vi "MAIN - PECT - Autonics - Pulses - encoder - stm32.vi"() -> ()   [LabVIEW 2018]
uses:
  Control 1.ctl
  <vilib>/DAQmx/read.llb/DAQmx Read (Counter U32 1Chan 1Samp).vi
  <vilib>/DAQmx/write.llb/DAQmx Write (Analog 1D Wfm NChan NSamp).vi
  <vilib>/DAQmx/read.llb/DAQmx Read (Analog 1D Wfm NChan NSamp).vi
  <vilib>/Instr/_visa.llb/VISA Configure Serial Port (Instr).vi
  <vilib>/DAQmx/create/channels.llb/DAQmx Create Channel (AI-Voltage-Basic).vi
  <vilib>/DAQmx/create/channels.llb/DAQmx Create Channel (CI-Count Edges).vi
  <vilib>/DAQmx/miscellaneous.llb/DAQmx Fill In Error Info.vi
  <vilib>/DAQmx/configure/timing.llb/DAQmx Timing (Sample Clock).vi
  <vilib>/DAQmx/configure/trigger.llb/DAQmx Start Trigger (Digital Edge).vi
  <vilib>/DAQmx/create/channels.llb/DAQmx Create Channel (AO-Voltage-Basic).vi
  LabViewtoPython/Global_data.vi
  <vilib>/measure/maspectr.llb/FFT Power Spectrum and PSD for 1 Chan.vi
  <resource>/objmgr/daqmx.rc
  <vilib>/Platform/NI_3dgraph.lvlib
  <vilib>/measure/NI_MAPro.lvlib
panel:
  in  "Filter 2":bool
  in  "low cutoff freq: fl 2":dbl=40.0 format="%0.2f"
  in  "Backdata":bool
  out "Numeric 2":i32=7858
  out "Init pulses":i32
  in  "Motor counter":tag="Dev3/ctr0"
  in  "Motor Counter Terminal":tag="PFI8"
  out "dy":dbl[][](array[numeric])
  in  "2D Array In":dbl[][](array[numeric])
  out "Output":dbl[][](array[numeric])
  out "Current  Position (mm)":dbl=12.5
  out "Acquire":bool=TRUE
  out "Numeric":dbl=22.0
  out "Enum":T1(ring)
  in  "Direction (+)":string="+"
  in  "Tab Control 3":enum32{"Control", "Data Processing"}(tab)
  in  "Encoder":bool=TRUE
  in  "Home":bool
  in  "Exit":bool
  in  "Scan":bool
  in  "Move Dis(mm)":dbl=150.0
  in  "Right":bool
  in  "Forward":bool
  in  "Left":bool
  in  "Backward":bool
  in  "Stop":bool
  in  "Pulser Trigger":tag="/Dev3/PFI0"
  in  "Edge":i32(ring)=10280 items=["Rising"=10280, "Falling"=10171]
  in  "2 Plots":bool
  in  "Offset":bool
  in  "Open csv":bool
  in  "Save Scan mode":bool caption="Save Process"
  in  "Gate 1":dbl
  in  "Gate 2":dbl=20.0
  in  "Open tdms":bool
  in  "Tab Control 4":enum32{"Basic", "Gaussian", "Chirp"}(tab)
  in  "Pulse Basic":T3={"Basic amp"=8.0, "Duty cycle %"=50.0, "Basic freq (Hz)"=200, "Basic Type"=2} {"Basic Type" items=["Sine Wave", "Triangle Wave", "Square Wave", "Sawtooth Wave"]; "Duty cycle %" format="%#.2f"; "Basic amp" format="%0.2p"}
  in  "Pulse Gaussian":T4={"Gauss amp"=2.8, "Gauss Nor. Band"=0.5, "Gauss atten (dB)"=6.0, "Gauss freq (Hz)"=1000.0}
  in  "Pulse chirp":T5={"Chirp amp"=2.1, "Chirp f2"=1500.0, "Chirp f1"=500.0} {"Chirp f1" format="%0.2f"; "Chirp f2" format="%0.2f"; "Chirp amp" format="%0.2f"}
  out "Motor Pulses":i32
  in  "Start idx":i32
  in  "End idx":i32=2000
  in  "Cursor":bool=TRUE
  in  "Repair Line Col":bool
  in  "Repair Line Row":bool
  in  "Line Col":dbl=167.0
  in  "Line Row":dbl
  in  "Y-max":dbl=55.0
  in  "Y-min":dbl
  in  "X-max":dbl=319.0
  in  "X-min":dbl
  in  "Inverse":bool caption="Scan"
  in  "ViewMode":i32(ring) items=["cwViewXYPlane", "cwViewXZPlane", "cwViewYZPlane", "cwViewUserDefined"]
  in  "Plot style":i32(ring)=5 items=["cwLine"=1, "cwPoint"=2, "cwLinePoint"=3, "cwHiddenLine"=4, "cwSurface"=5, "cwSurfaceLine"=6, "cwSurfaceNormal"=7, "cwContourLine"=8, "cwSurfaceContour"=9]
  in  "ColorMapAutoScale":bool=TRUE
  in  "Max":dbl=0.6
  in  "Min":dbl=-0.8
  in  "low cutoff freq: fl":dbl=40.0 format="%0.2f"
  in  "Filter":bool caption="Scan"
  in  "Backindex":i32
  in  "Backdata":bool caption="Scan"
  in  "Odd":bool caption="Scan"
  in  "DiffX":bool caption="Scan"
  in  "DiffY":bool caption="Scan"
  in  "Abs":bool caption="Scan"
  in  "Trim data":bool caption="Scan"
  in  "Return":bool caption="Scan"
  out "No.data":i32
  in  "Tab Control 2":T6(tab)
  out "Hall sensors signal":waveform(dbl)[](graph)=[{"t0"=timestamp(3772601412.9474645 s since 1904-01-01), "dt"=9.999999999999972e-06, "Y"=array[500 elements], "attributes"=variant("NI_ChannelName"=variant(string "Acquisition Task0"), "NI_UnitDescription"=variant(string "Volts"))}, {"t0"=timestamp(3772601412.9474645 s since 1904-01-01), "dt"=9.999999999999972e-06, "Y"=array[500 elements], "attributes"=variant("NI_ChannelName"=variant(string "Acquisition Task0"), "NI_UnitDescription"=variant(string "Volts"))}]
  out "Feature Extraction":dbl(graph)=9.808813079931117
  out "Power spectral density":cluster{"f0":dbl, "df":dbl, "magnitude":dbl[]}[](graph)=[{"f0"=0.0, "df"=200.00000000000054, "magnitude"=[0.014362964529831107, 8.310174695746657, 3.5091233603848444, 0.7631604563682475, 0.42177215625270154, 0.19736118568021033, 0.12192952566419618, 0.06836206987142136, 0.04491682851594746, 0.027429593107677796, 0.018839071574379328, 0.012148402422180482, 0.00862941575502791, 0.005816349612651425, 0.004256233122154165, 0.0029703985982499756, 0.00222866785183307, 0.001605169236331863, 0.0012333117661796167, 0.0009173667056733339, 0.0007155423005092866, 0.0005404107405385125, 0.00042969027524349985, 0.000330389538775732, 0.00026610143624204957, 0.00021016892953679833, 0.00017149707496417528, 0.0001376562085986954, 0.00011376018152653006, 9.192625603438476e-05, 7.690968629569889e-05, 6.331696380512943e-05, 5.369944415943588e-05, 4.483264313157133e-05, 3.783661085972104e-05, 3.171641922275525e-05, 2.7287859659355045e-05, 2.2939811822779873e-05, 1.9729023645397208e-05, 1.6853998605376913e-05, 1.4418164836398328e-05, 1.2221148062729234e-05, 1.0824528543421417e-05, 9.63348776166626e-06, 8.38664900977408e-06, 7.088182653208775e-06, 6.4216695750381725e-06, 5.838100076590925e-06, 5.062973197813572e-06, 4.380481399910079e-06, 4.008311134417931e-06, 3.567777110785873e-06, 3.1057220585572244e-06, 2.7147559678671816e-06, 2.469004683700486e-06, 2.2349741034633414e-06, 1.9591588689462376e-06, 1.6850457298246318e-06, 1.4830403711511327e-06, 1.2810395862247023e-06, 1.1661807691347021e-06, 1.093149967617751e-06, 1.0079255280756182e-06, 9.738198789620943e-07, 9.715762489409555e-07, 8.96196851562932e-07, 7.523554510993729e-07, 6.138187229264334e-07, 5.478503267370196e-07, 5.020387710315625e-07, 4.619114100892691e-07, 4.2419919587483664e-07, 3.871191758999957e-07, 3.3109894129644344e-07, 2.7247124240836894e-07, 2.4850669965307075e-07, 2.675581974815067e-07, 2.869535576611872e-07, 2.7749898679948705e-07, 2.4632291660033263e-07, 2.1801622453669157e-07, 1.9562127404410693e-07, 1.7794867931791103e-07, 1.6811228641885276e-07, 1.5616631012591995e-07, 1.2698956764184784e-07, 1.1852206215172555e-07, 1.4052784440882626e-07, 1.2417001647212458e-07, 1.0284765504537362e-07, 1.1149589035952914e-07, 1.0511333967341304e-07, 8.631594494061448e-08, 7.61357409684589e-08, 6.937531533687657e-08, 7.010901044974718e-08, 8.376351369143556e-08, 8.332819916917156e-08, 7.575462195169617e-08, 7.885454530850919e-08, 7.033884155079282e-08, 6.000608335599921e-08, 5.97054760945729e-08, 5.485461457908942e-08, 4.5798277681414524e-08, 3.8358139340699667e-08, 3.3676177145198874e-08, 2.359178779533516e-08, 1.8510156950926208e-07, 5.633600043987599e-07, 1.2855680539466263e-07, 1.678757147241346e-09, 9.284437562813088e-09, 1.0545287775390088e-08, 1.4885830217932153e-08, 2.288209497269105e-08, 2.873109268361236e-08, 3.240059456948882e-08, 2.9373366158461235e-08, 1.6941482060852982e-08, 1.3632670056174659e-08, 2.1599039524822428e-08, 2.864941019474429e-08, 2.6325731881126113e-08, 1.7196134685578826e-08, 1.285975985125537e-08, 2.487391402547663e-08, 3.203240697565154e-08, 1.720084880141038e-08, 1.198157151831842e-08, 4.459277430827087e-08, 3.303106142973774e-08, 2.133721419654825e-09, 5.109784879397802e-09, 1.3424442340069317e-08, 1.6867214043579696e-08, 1.5794232523657268e-08, 1.5127476306279365e-08, 1.5161128228270264e-08, 1.6118426952093236e-08, 1.68634299672962e-08, 1.6945853543588977e-08, 1.6868974698788065e-08, 1.0784883043928202e-08, 6.704461125465945e-09, 5.63854300858233e-09, 5.0266424135467835e-09, 6.568105272929862e-09, 7.59825171358279e-09, 1.1582490374347768e-08, 1.4599621166870617e-08, 1.1119981753358133e-08, 1.2942473625642193e-08, 1.774060483085851e-08, 1.2500855965824921e-08, 6.798673179813089e-09, 3.825701426335919e-09, 3.26796645153504e-09, 5.851436091197948e-09, 9.117713523866911e-09, 1.006129981484824e-08, 9.670570433095903e-09, 6.903128148171139e-09, 4.6017756529415e-09, 5.3985244057071846e-09, 5.091422999856316e-09, 6.324668231652877e-09, 1.2737016312662349e-08, 1.1044421774333567e-08, 8.651162714385546e-09, 1.1322218007796528e-08, 2.001816258965483e-08, 5.928473615592085e-09, 7.891019427142181e-08, 2.710947551074279e-08, 1.2109707937657889e-08, 1.5145237102579988e-08, 5.528097117459409e-09, 2.446227470013534e-09, 4.474934593714336e-09, 5.0407366988498425e-09, 3.111049069643071e-09, 2.815789099676651e-09, 2.198647691132389e-09, 3.564152929351252e-09, 6.267856744894125e-09, 7.855009262955687e-09, 7.797377233153132e-09, 4.960163939861098e-09, 4.126978597434626e-09, 7.818217929097502e-09, 1.2088488517836051e-08, 1.5807096200904325e-08, 1.4005329604816694e-08, 5.851220743643767e-09, 2.6117978983188714e-09, 2.109976569403879e-09, 5.079632540665155e-09, 1.4259080894475479e-08, 1.495379496959781e-08, 9.052261543456204e-09, 3.575730290321285e-09, 3.1053726421904294e-09, 4.820372466465575e-09, 4.369001562192545e-09, 3.7977013602532216e-09, 6.3454386055254605e-09, 6.575277240465807e-09, 5.475129294692274e-09, 5.322703673955227e-09, 5.009070823464934e-09, 4.896565904493876e-09, 6.143932752088867e-09, 5.958661103676973e-09, 7.581104983628496e-09, 1.29243222401234e-08, 1.639764632220392e-08, 1.62303693108852e-08, 1.4889908382954265e-08, 6.265747183052516e-09, 3.5369901111449913e-09, 3.99415669353274e-09, 4.336446347036391e-09, 5.2993261898260645e-09, 7.707397886429536e-09, 6.012570048278088e-09, 5.397447185281157e-09, 6.015860855807052e-09, 4.357450363448522e-09, 7.100715289952546e-09, 9.805560081159733e-09, 6.950732862283354e-09, 6.8841271181353234e-09, 4.007604528286423e-09, 2.256008744538429e-09, 4.9771864801295934e-09, 8.071283941533974e-09, 4.167385572741655e-09, 1.6583946978149515e-09, 4.0472343516843064e-10, 8.66146004461999e-09, 6.3560460604905285e-09, 1.133124355330132e-09, 3.296374300658255e-09, 1.0980369368354793e-08, 1.459727038058513e-08, 1.3676634631114127e-08, 8.996399934605576e-09, 6.0440593342303344e-09, 7.04368222367538e-09]}, ...(2 in all)]
  in  "Add LF":bool
  in  "Save LF":bool caption="Save Process"
  in  "3D Surface":refnum<k7>(container)
  out "Record path":path=path "G:/Shared drives/ICSLab-Students/NDT/PECT/Data/Scan NewBoard/PECT_default.tdms" caption="selected path"
  out "Feature extraction scan":dbl[](graph)
  in  "View Mode":bool caption="Scan"
  out "Hall sensors signal lf":dbl[][](graph)=[[-0.70660846198, -0.716567731313, -0.71772803455, -0.717921418426, -0.720596562008, -0.722079171705, -0.724657623384, -0.723561781416, -0.729298836376, -0.728847607304, -0.733553281611, -0.731232675116, -0.734068971955, -0.734230125187, -0.734649123582, -0.735197044564, -0.737292036575, -0.735906118769, -0.738162264033, -0.736454039766, -0.735454889741, -0.737968880154, -0.735422659102, -0.737292036581, -0.734552431644, -0.735809426849, -0.731909518652, -0.731264905752, -0.726591462081, -0.727171613726, -0.72340062815, -0.721080021693, -0.715278505501, -0.71253890069, -0.707188613582, -0.701870557272, -0.697068191179, -0.692362517146, -0.687946918849, -0.677826496722, -0.674571201711, -0.663773936246, -0.660776486438, -0.651622983945, -0.644113244288, -0.636120045089, -0.629867300614, -0.618425422989, -0.610399993434, -0.59950603696, -0.59218968167, -0.58322956384, -0.571207535404, -0.564471331877, -0.553126147145, -0.546615558225, -0.534915836753, -0.528792015616, -0.520315358066, -0.514803919133, -0.504103347861, -0.497753912499, -0.490534250062, -0.48415258421, -0.4781254554, -0.472839631231, -0.469197569495, -0.467811652195, -0.46571666097, -0.462429136198, -0.467457115235, -0.467231500771, -0.474354471106, -0.474741238726, -0.482927820085, -0.490469788806, -0.499204291135, -0.509066865834, -0.523216115386, -0.534432377128, -0.554350911396, -0.569177005115, -0.58816085171, -0.612366062487, -0.634250667901, -0.66187232831, -0.688269225307, -0.719081721676, -0.746928999864, -0.781093486223, -0.813130751347, -0.851227380515, -0.888357092222, -0.928000797226, -0.965807357181, -1.008351826422, -1.048994689492, -1.09189370194, -1.13485717869, -1.180109036257, -1.2251352826, -1.266293851833, -1.314639865003, -1.35380013893, -1.401147008934, -1.441370901989, -1.48307740981, -1.522592234217, -1.561881446939, -1.594208832793, -1.628276678402, -1.656575231322, -1.685228323683, -1.708627813295, -1.726709237842, -1.745338585167, -1.754749951221, -1.765386084343, -1.766481928394, -1.766578620469, -1.759068865834, -1.749141808352, -1.726870391409, -1.702697363978, -1.672142659225, -1.635496354594, -1.591855992024, -1.542736415895, -1.486816169566, -1.426544787201, -1.357119898907, -1.281152192711, -1.205055574576, -1.115615471107, -1.027496838527, -0.924487655795, -0.823476790057, -0.71266782326, -0.598377964549, -0.477738687781, -0.356454816131, -0.226146385508, -0.096933813379, 0.039691785785, 0.177477671952, 0.315553620416, 0.456562543074, 0.59605661768, 0.738386978448, 0.878138885599, 1.019921318004, 1.154935322631, 1.292076548544, 1.418613908244, 1.546504957955, 1.665822671713, 1.781143796386, 1.887472587349, 1.990352709737, 2.080759590593, 2.164752584475, 2.235692182322, 2.298122899903, 2.352689348501, 2.387788500997, 2.419503438832, 2.429204857999, 2.432524612792, 2.418181983039, 2.390753718718, 2.346694452024, 2.29477091497, 2.222380935278, 2.137904477937, 2.035346650361, 1.920347813654, 1.791425361517, 1.644195932762, 1.485299034053, 1.310738069287, 1.125154243505, 0.921650202866, 0.71092650171, 0.483765177519, 0.253445229601, 0.008105779367, -0.246129373952, -0.508261099919, -0.779449723152, -1.058244889529, -1.341584711586, -1.635528585329, -1.928441259944, -2.223868134907, -2.526772774422, -2.823650514512, -3.124106146674, -3.41405481644, -3.706227714753, -3.987442417835, -4.263822791101, -4.527407776882, -4.786577416573, -5.02840704592, -5.262275871216, -5.475098028081, -5.677574208879, -5.860454027961, -6.026509320014, -6.174450790588, -6.300217254762, -6.406645020668, -6.487352250666, -6.552781862445, -6.587011551361, -6.605834660103, -6.593973522799, -6.560743004097, -6.502017506172, -6.420568948967, -6.309918874295, -6.178350774499, -6.019772990024, -5.841921080871, -5.636479455639, -5.407702708707, -5.163100759281, -4.889329996495, -4.60340849308, -4.29102572782, -3.966589007543, -3.624329025262, -3.267791211866, -2.894429352616, -2.512784620922, -2.118957082525, -1.720230866355, -1.310095339563, -0.893610688781, -0.473226398891, -0.047749885035, 0.377081857903, 0.806651402224, 1.226326113266, 1.646645459066, 2.057327931374, 2.465367624173, 2.856937640696, 3.240772514315, 3.608041067282, 3.955230157274, 4.293975068757, 4.609804197942, 4.90271751193, 5.177098363499, 5.426887322034, 5.649860408204, 5.851142279943, 6.021772700426, 6.172194436626, 6.288354759714, 6.38169561436, 6.443353457295, 6.479452149573, 6.483029788153, 6.46127387881, 6.407834927929, 6.330674003129, 6.221217696105, 6.086943623705, 5.925176659162, 5.736206928573, 5.524965806055, 5.286167477957, 5.029771319924, 4.744593282131, 4.446168641795, 4.123506733751, 3.788113950506, 3.432351621052, 3.06650133258, 2.685180548865, 2.296898136162, 1.899107838935, 1.494871524426, 1.086445286821, 0.675762909712, 0.265467248353, -0.150952337452, -0.55870204758, -0.972221258056, -1.373654237756, -1.777923829368, -2.168979184481, -2.552460698049, -2.920729689806, -3.280071163481, -3.622008401497, -3.950860315772, -4.258117910152, -4.550936409787, -4.823256343074, -5.072595856712, -5.304498634402, -5.509682053404, -5.698202166799, -5.859132548236, -6.000240858013, -6.111889905191, -6.206424214181, -6.27008099717, -6.315365963394, -6.333898960157, -6.329676659853, -6.305148642671, -6.25857442753, -6.185216035338, -6.09506518857, -5.986381425725, -5.856360663809, -5.709708700472, -5.54117189352, -5.365641079165, -5.166356100054, -4.957401996174, -4.734878834588, -4.502332058483, -4.25769890765, -4.007715673153, -3.745098175872, -3.482835479658, -3.212193012196, -2.937618633024, -2.664784953904, -2.386601188071, -2.116185239442, -1.843835631437, -1.575257184583, -1.307226809354, -1.048865766862, -0.789924683906, -0.543553647601, -0.298858680926, -0.065186650983, 0.160975596988, 0.377855392589, 0.583937909112, 0.777321550784, 0.961906228802, 1.129988834268, 1.286113886493, 1.434406905534, 1.559977352138, 1.681841284773, 1.782239637185, 1.87196966226, 1.947711605492, 2.009916693762, 2.057166778279, 2.095037754511, 2.114505048262, 2.126913836672, 2.123561852274, 2.106834160961, 2.083724807448, 2.04517698859, 1.999828510872, 1.941362174369, 1.876127411384, 1.800417702224, 1.720518017024, 1.626759173182, 1.53477301667, 1.432666452766, 1.3256930704, 1.216753623473, 1.100658983649, 0.982533816097, 0.864892106737, 0.741448886061, 0.618489120633, 0.497011957912, 0.371215886709, 0.252865078568, 0.127455756566, 0.00929831228, -0.108053378055, -0.221569636608, -0.333216531681, -0.440351151746, -0.547066787125, -0.643984321714, -0.742481170629, -0.834016212751, -0.919943133402, -1.004129610016, -1.078743591058, -1.154131117554, -1.220526296559, -1.28176457554, -1.335299729295, -1.389318348703, -1.430928160202, -1.472151206875, -1.504381894686, -1.533711822363, -1.557723687612, -1.576417489536, -1.58798830868, -1.597464132915, -1.601750815379, -1.601621892616, -1.59852774587, -1.588246154234, -1.580027327232, -1.560882295453, -1.54560494743, -1.52268892626, -1.50177120885, -1.474117278751, -1.447236886611, -1.415296278632, -1.385869665753, -1.349996918726, -1.315800169399, -1.280926577982, -1.245472836775, -1.210728172549, -1.170472066246, -1.137048863988, -1.097276222791, -1.065400096546, -1.027077839927, -0.994814949512, -0.958942227201, -0.927646259992, -0.892128078709, -0.861283343899, -0.830664225057, -0.801817793355, -0.772777978979, -0.746928999873, -0.722723784605, -0.697132652466, -0.677504190288, -0.654072512801, -0.640019952773, -0.620713798494, -0.607112468066, -0.589804614323, -0.577589201926, -0.565986171871, -0.555930212629, -0.54590648416, -0.539105819592, -0.533239843546, -0.528050710938, -0.523635113662, -0.51996082103, -0.521346738438, -0.518703826188, -0.521314507795, -0.519896359761, -0.525472259972, -0.524408648935, -0.530177933006, -0.532079540602, -0.538815743842, -0.541813193149, -0.548871702871, -0.55319060837, -0.559572274784, -0.565953941223, -0.570885229012, -0.57865281302, -0.584647711969, -0.594349134521, -0.597120969574, -0.607305851908, -0.611399143265, -0.6213584113, -0.626902081599, -0.634282898507, -0.640019952747, -0.647046232714, -0.651300677507, -0.657295577056, -0.662162404096, -0.668737455294, -0.674216664635, -0.675602582331, -0.683531320648, -0.684949468998, -0.693136052559, -0.694167433224, -0.700516870141, -0.703095321724, -0.708961299059, -0.708219994242, -0.711443058732], [-0.711700903907, -0.720274255531, -0.721080021681, -0.724464239466, -0.722433708801, -0.725141083016, -0.72559231207, -0.726204694336, -0.729202144406, -0.727848457275, -0.731039291205, -0.729975679907, -0.73139382833, -0.73123267509, -0.734165663872, -0.732392978358, -0.735648273607, -0.732908668699, -0.73590611877, -0.734810276807, -0.73352105101, -0.733843357422, -0.732844207425, -0.733230975136, -0.731007060611, -0.73062029283, -0.728106302452, -0.729427758908, -0.724174163692, -0.726043541112, -0.72166017329, -0.721208944256, -0.715181813577, -0.712248824884, -0.70754315068, -0.704739084581, -0.697809495981, -0.693361667074, -0.688849376879, -0.681694173927, -0.676311656471, -0.666481310252, -0.663677244331, -0.654942740122, -0.649270147063, -0.638827419012, -0.632703597094, -0.62161625644, -0.613816441327, -0.601891104324, -0.593382215333, -0.583906407255, -0.574301676729, -0.564729176965, -0.553480684115, -0.54616432927, -0.535624910724, -0.527373867557, -0.517382370077, -0.511258549117, -0.498881984754, -0.493789544277, -0.484603813104, -0.479898140329, -0.472710708686, -0.46910087758, -0.464072898546, -0.462042368558, -0.459721762867, -0.45836807625, -0.458948227649, -0.460366375577, -0.465104278851, -0.467167039506, -0.476352770465, -0.481703055936, -0.495368845435, -0.504619038035, -0.520702125685, -0.534819144789, -0.554447603261, -0.570530691961, -0.592511988075, -0.615621357208, -0.640535643041, -0.667319306976, -0.694973199311, -0.727912918571, -0.7584675715, -0.795017126404, -0.828988231267, -0.870404618505, -0.908050021807, -0.951432484146, -0.989754736086, -1.033685125354, -1.077228749861, -1.121674836208, -1.166572155322, -1.211276093955, -1.257140340429, -1.302521130597, -1.347934155322, -1.389930731637, -1.437535450536, -1.478565113577, -1.521947620419, -1.557949302468, -1.598431053803, -1.629565906268, -1.663762677273, -1.691223234113, -1.718941638241, -1.740310595099, -1.759874633465, -1.772831377568, -1.782081590668, -1.788237655914, -1.788173194541, -1.784176586682, -1.7728636083, -1.758134175287, -1.733090917251, -1.706693971085, -1.669886510205, -1.632917898781, -1.584314009521, -1.53206805716, -1.471442131748, -1.407141915873, -1.333398119264, -1.254561886613, -1.168796071461, -1.07871136044, -0.983147451101, -0.877076363675, -0.77200444347, -0.655490661079, -0.541426425506, -0.414760028952, -0.290317564379, -0.158687687189, -0.026832212351, 0.113370977212, 0.253509690839, 0.395968995891, 0.538202675996, 0.682209031094, 0.82640876359, 0.965999515658, 1.107943100394, 1.2432149505, 1.379195876537, 1.506635696159, 1.632560682823, 1.748236342269, 1.865201233481, 1.969338348306, 2.067416114716, 2.15692054372, 2.236530178481, 2.30560040478, 2.364485757723, 2.409930942223, 2.44470779056, 2.468332842109, 2.474327739345, 2.470137757407, 2.448124237269, 2.417408447956, 2.366355134083, 2.304955792292, 2.22576515062, 2.134197956683, 2.022454403625, 1.899978065497, 1.759420364327, 1.606872887466, 1.438564653815, 1.256074962083, 1.059951729476, 0.851161868759, 0.630478906609, 0.399030903911, 0.159009529445, -0.095741280337, -0.355101129604, -0.628997073303, -0.906148413194, -1.193065765257, -1.484979020361, -1.782984050494, -2.083052046727, -2.385956572993, -2.689473733606, -2.994473784422, -3.295767585382, -3.589680826897, -3.885270392832, -4.167097682705, -4.447442674322, -4.711382413403, -4.969939881134, -5.21305896681, -5.445155293591, -5.65475453306, -5.853298698642, -6.032053093797, -6.193563935177, -6.333222102904, -6.451672172544, -6.551138064005, -6.625721405834, -6.678709764359, -6.705397338156, -6.7118436127, -6.689732892102, -6.647219721964, -6.571991743565, -6.476812606234, -6.354849306761, -6.207552308847, -6.03563076211, -5.840825219647, -5.620911798473, -5.380693017663, -5.114625193963, -4.828993469243, -4.526666463854, -4.200843492433, -3.861516208625, -3.502302924475, -3.13216385381, -2.744427224852, -2.350406050506, -1.943944235937, -1.534034129331, -1.111328792601, -0.688108072092, -0.254348183817, 0.180185043615, 0.614653678333, 1.048574325895, 1.479626447166, 1.903394510606, 2.321264488474, 2.731753822843, 3.124806592014, 3.511768013492, 3.874782309212, 4.221391454251, 4.556655670645, 4.868101642753, 5.155503714809, 5.423470852265, 5.66481553335, 5.882245096744, 6.070795930585, 6.233626609533, 6.371091627426, 6.475326584487, 6.555807348401, 6.601285277357, 6.622976737884, 6.609955415071, 6.570891451368, 6.499628742443, 6.407544849292, 6.28052263845, 6.128070288235, 5.948608528303, 5.743491108137, 5.514426315553, 5.258964657354, 4.982101962969, 4.683548195569, 4.366655388863, 4.026975726542, 3.675113132109, 3.302687625615, 2.924912076204, 2.52876527563, 2.127365065353, 1.717166033533, 1.303228338131, 0.883199090654, 0.465587113791, 0.041722314718, -0.374858506392, -0.792632058415, -1.209664560433, -1.619703313065, -2.022973968836, -2.416640254231, -2.801153418931, -3.170164003204, -3.529376856542, -3.867414465728, -4.195654308351, -4.499141189584, -4.786964188961, -5.051871271029, -5.297149939141, -5.518352233991, -5.717154105289, -5.893104251006, -6.046299304766, -6.173645008773, -6.275238003521, -6.35791128069, -6.408675593623, -6.444194505839, -6.448062264612, -6.433687095446, -6.394268196495, -6.335252674733, -6.248389341404, -6.145345955566, -6.020353152397, -5.879180364564, -5.71757311064, -5.538109933487, -5.346721406584, -5.136058870085, -4.916694164197, -4.681472020658, -4.438804768894, -4.185340402521, -3.926783816261, -3.653465746224, -3.381437188134, -3.103252801735, -2.823908360859, -2.542275774546, -2.258999645662, -1.980912873448, -1.705791511432, -1.431605004604, -1.161544171119, -0.901281584442, -0.641986021923, -0.394615883648, -0.147374738228, 0.083364272888, 0.312008253063, 0.526470734451, 0.730973938979, 0.921811355892, 1.10391427476, 1.267806902505, 1.422997270747, 1.563135951752, 1.687868408833, 1.801094545084, 1.89701284902, 1.981811596561, 2.050430579225, 2.106834160953, 2.147799278231, 2.17816052264, 2.190633772981, 2.194823753727, 2.183317421989, 2.162238596067, 2.128299753321, 2.084208266714, 2.0311889008, 1.967017743996, 1.893370789696, 1.81256864297, 1.725739375948, 1.627307093536, 1.528359125728, 1.41655114942, 1.30799846779, 1.188100615371, 1.068557301022, 0.944695085629, 0.822992319382, 0.695069043221, 0.570272131299, 0.442284382926, 0.317616379586, 0.194624359058, 0.068441497018, -0.050553949051, -0.171128708146, -0.285160663856, -0.399676092901, -0.508132177389, -0.615073436322, -0.712184363585, -0.810874605876, -0.899960127607, -0.986692823527, -1.067462858994, -1.142721461342, -1.214112393046, -1.278251431973, -1.337298031367, -1.389382810045, -1.440339520092, -1.481240260618, -1.520884007654, -1.548602401773, -1.57802902429, -1.595723675412, -1.612902636098, -1.621959461795, -1.628502293261, -1.629275830005, -1.627986602099, -1.618188470277, -1.608358107981, -1.59524021497, -1.575482799408, -1.556627844048, -1.531455674043, -1.507895039751, -1.477243655394, -1.44794596169, -1.414168204733, -1.38277552038, -1.345710238439, -1.31270602436, -1.274061444278, -1.238059782054, -1.200704434038, -1.16164086315, -1.124865672142, -1.086188874377, -1.050283915983, -1.013218656049, -0.978731850936, -0.941376519413, -0.91175654708, -0.874530142074, -0.846586166678, -0.814258824097, -0.786379312543, -0.757500652045, -0.731554981564, -0.705641542641, -0.684433778674, -0.659003801079, -0.639955491476, -0.622712098238, -0.603212560587, -0.590352535192, -0.573463680108, -0.562601954829, -0.551933613494, -0.542554497827, -0.532853075905, -0.529694473448, -0.52025089677, -0.519058363199, -0.513837000046, -0.511451932947, -0.512870080968, -0.511838700566, -0.511677547393, -0.514352690234, -0.517285678205, -0.520508741861, -0.526568101624, -0.527825096497, -0.538493437484, -0.540427275726, -0.547389093516, -0.553061685838, -0.559540044149, -0.566147325069, -0.57620328444, -0.578652813016, -0.588676541915, -0.596540818049, -0.602116718805, -0.61207598672, -0.616749429656, -0.626450852631, -0.6339605921, -0.639955491487, -0.645563623199, -0.654459280486, -0.657263346399, -0.666739155394, -0.66922091493, -0.67573150487, -0.681823096537, -0.68501393027, -0.690783215552, -0.69532773638, -0.698035110534, -0.70357878138, -0.706382847481, -0.706995229747, -0.714827276494, -0.711829826488, -0.717115652296], [-0.710927368415, -0.721563481368, -0.721595712031, -0.723303936229, -0.725108852432, -0.725527850816, -0.729427758978, -0.727300536363, -0.732876438089, -0.733166513892, -0.737034191399, -0.735003660722, -0.738549031766, -0.738452339841, -0.737968880135, -0.738903568875, -0.741095252863, -0.738645723707, -0.741030791566, -0.739677104411, -0.739354797941, -0.742094402897, -0.73774326562, -0.742932399702, -0.737743265618, -0.738968030203, -0.735519351038, -0.735035891386, -0.730845907349, -0.72978229604, -0.724464239482, -0.723819626589, -0.716019810351, -0.714408278121, -0.708574531326, -0.703063091172, -0.698679723421, -0.692878207473, -0.688398147883, -0.678213264461, -0.674829046864, -0.664257395879, -0.659519491377, -0.650656064667, -0.642179405778, -0.633799438886, -0.625226088263, -0.614525515429, -0.606081087604, -0.593478907265, -0.587516238926, -0.577041281088, -0.564471331913, -0.558605355655, -0.545197410173, -0.540781812775, -0.528276325465, -0.521250046516, -0.512773389061, -0.505295881372, -0.496013458178, -0.490598711337, -0.480768367493, -0.477255228246, -0.470325641713, -0.466393504254, -0.46226798305, -0.458819305132, -0.460559759439, -0.456659852641, -0.462429136215, -0.463879514767, -0.471389252665, -0.472517324904, -0.483153434512, -0.490502019438, -0.50084805357, -0.513160156676, -0.528147402851, -0.542361113995, -0.561699496934, -0.579780885408, -0.602664639692, -0.627611155718, -0.650108143758, -0.682467709413, -0.707704303918, -0.742610093227, -0.773390361308, -0.810391146154, -0.844877942157, -0.884070415338, -0.922714969748, -0.965130513384, -1.004194071312, -1.050251685316, -1.092699468449, -1.135695176079, -1.183235411066, -1.227133584269, -1.276382052832, -1.317637317973, -1.366466795995, -1.408012144306, -1.454714405619, -1.494777149486, -1.537934042904, -1.57635302815, -1.614095171865, -1.647905173327, -1.679620181747, -1.706984047416, -1.734025607719, -1.755845795159, -1.771058688734, -1.787077350425, -1.793910260671, -1.803063782041, -1.796939947333, -1.794844951197, -1.782500589886, -1.765353853546, -1.740826286392, -1.711657499304, -1.673367425821, -1.633207975063, -1.581703323307, -1.527845836705, -1.464705918282, -1.396151253222, -1.324856989698, -1.238930010223, -1.155291421567, -1.061242341096, -0.964228054985, -0.855095058719, -0.747960380555, -0.628481383047, -0.509260249656, -0.382271551645, -0.252317654314, -0.117787026094, 0.01909642047, 0.16013760098, 0.300663077532, 0.445829750017, 0.592833556893, 0.73248877748, 0.882199941889, 1.021210542207, 1.165829267176, 1.303453952372, 1.438274578348, 1.570484530423, 1.696796287823, 1.813857867449, 1.930307073514, 2.031124439534, 2.130330282341, 2.219673563048, 2.293578381865, 2.362261844503, 2.416119222821, 2.462434636828, 2.491828971774, 2.511876424447, 2.513326802871, 2.507525289189, 2.480902787945, 2.44390202482, 2.389980183652, 2.321103335349, 2.237626019648, 2.138613551575, 2.020552797226, 1.892371640636, 1.746141352558, 1.583860232908, 1.41087856266, 1.216528009233, 1.019792395584, 0.801139968617, 0.572592735082, 0.334891987588, 0.086426181539, -0.174448462454, -0.439416463364, -0.719307336175, -1.001099928024, -1.292304006338, -1.591630377162, -1.893019701465, -2.201209923647, -2.506660775153, -2.815625046101, -3.122430143612, -3.429364475269, -3.72505055753, -4.023057597177, -4.307076750992, -4.584972354295, -4.851974206402, -5.106148417387, -5.347559415797, -5.576948483823, -5.784839614889, -5.981159965478, -6.156111198496, -6.30959656147, -6.45041515099, -6.55987275788, -6.655793263995, -6.722995668099, -6.76869976497, -6.787490663209, -6.783590665282, -6.752519610718, -6.698564287283, -6.615794148269, -6.511880294189, -6.378281466584, -6.220025813415, -6.041238998862, -5.833121960323, -5.605054062077, -5.350234599383, -5.079590001991, -4.780034515432, -4.468360588381, -4.130322168267, -3.780036472621, -3.411089577322, -3.030185528628, -2.634907020607, -2.231700205315, -1.816117219547, -1.398761938448, -0.967870119262, -0.533948917579, -0.10031802868, 0.342014952778, 0.778997542299, 1.221878289721, 1.653542809478, 2.083595884971, 2.502368388148, 2.912342123176, 3.308199069955, 3.69280778213, 4.05759490835, 4.402173670004, 4.736986818805, 5.045499953056, 5.330420413114, 5.590007684748, 5.831030201483, 6.037340233968, 6.223796171648, 6.375088266782, 6.505817090897, 6.600028268508, 6.67061415748, 6.707615353626, 6.71873505223, 6.697236968676, 6.649148309384, 6.567990662195, 6.460919338063, 6.323744347412, 6.159398755148, 5.970042083259, 5.748390202495, 5.509785072288, 5.239207160015, 4.951933935452, 4.638650733591, 4.311863128522, 3.962482067337, 3.598823090781, 3.219435814265, 2.828187905105, 2.423532267353, 2.013268677874, 1.593787260336, 1.170857241583, 0.745058713974, 0.317455226524, -0.10628069381, -0.536559599228, -0.956170390698, -1.37877891595, -1.790010344895, -2.197890157421, -2.592974779821, -2.979196378686, -3.349786489195, -3.70845164637, -4.045715944667, -4.3717965508, -4.673607650656, -4.956273909006, -5.2199564235, -5.459272535097, -5.679089074392, -5.868286213282, -6.041658005013, -6.18408794079, -6.30775937747, -6.402938419599, -6.474846495158, -6.520550523301, -6.54420832557, -6.539824863307, -6.514362106984, -6.463887844289, -6.3946872037, -6.301667662811, -6.18431355981, -6.054260422905, -5.897584390787, -5.732012684015, -5.54088181332, -5.340758648073, -5.123682130552, -4.894293578911, -4.649466615545, -4.398161494277, -4.134189881976, -3.865738458211, -3.588165975379, -3.308531000887, -3.0243839815, -2.736756297111, -2.452932090653, -2.16456357347, -1.884962022521, -1.602911120461, -1.331432047928, -1.056794509731, -0.793631208497, -0.533046459727, -0.280068224611, -0.036372475961, 0.196300351006, 0.424912084094, 0.636344877161, 0.841073689194, 1.031073107354, 1.206472060374, 1.373845595888, 1.519656861632, 1.659795547723, 1.778468655645, 1.889341962949, 1.981070292399, 2.061356758571, 2.12433538713, 2.176226685399, 2.211293601344, 2.236240102863, 2.244781217885, 2.243040764236, 2.228472522925, 2.201495492363, 2.160498142613, 2.110605143374, 2.055104018764, 1.981038061762, 1.907165492431, 1.816758622552, 1.72515922494, 1.623342728618, 1.517207335446, 1.405012592267, 1.290142712201, 1.168246562564, 1.047156179274, 0.919039523837, 0.792727780462, 0.665803652141, 0.534979615125, 0.407733168748, 0.276586809842, 0.152950173688, 0.024575625662, -0.097675117694, -0.219539107163, -0.33276530288, -0.44750635248, -0.555833520716, -0.659648413935, -0.759434490888, -0.85722228175, -0.945888811272, -1.032557052242, -1.113939476566, -1.187393167446, -1.260202254478, -1.321988459376, -1.383935824916, -1.431895080745, -1.481530336808, -1.52059393143, -1.554532849089, -1.584926392742, -1.610227488406, -1.62624614447, -1.64239372398, -1.647872942625, -1.65280423958, -1.652836470222, -1.645584563108, -1.639911960213, -1.625472607776, -1.610549795346, -1.5874726176, -1.567940817251, -1.540705882338, -1.514212254869, -1.483045179111, -1.452554949714, -1.416521044576, -1.38277552039, -1.345001163501, -1.307291270799, -1.268163230894, -1.23274172125, -1.193581455997, -1.150585744158, -1.117291465704, -1.074875911501, -1.041484945369, -1.003001536946, -0.967515582024, -0.932223013107, -0.898219672272, -0.863507258885, -0.833178215835, -0.799142649494, -0.772745748364, -0.743351398115, -0.716471039411, -0.693587281637, -0.668092842444, -0.650688295345, -0.627256618724, -0.612881752772, -0.595863974652, -0.583519639569, -0.56724316682, -0.556800439871, -0.545551947147, -0.535721602628, -0.528276325388, -0.523796266856, -0.516060913979, -0.514094845139, -0.511065165314, -0.508841251385, -0.512032084435, -0.509002404553, -0.516350989715, -0.514513843417, -0.520831048233, -0.522764886451, -0.526729254832, -0.53195061806, -0.538590129407, -0.541652039967, -0.550966694366, -0.553802990491, -0.563053183779, -0.569853848527, -0.575590902357, -0.584905557093, -0.590932686735, -0.601020877055, -0.60350263635, -0.614944513774, -0.618908882582, -0.629125995866, -0.634927511342, -0.643146325024, -0.647884229412, -0.655651814247, -0.659551722015, -0.665675544213, -0.668963069777, -0.677633112898, -0.681629712678, -0.682854477157, -0.691717904228, -0.692169133285, -0.701097021755, -0.701580481458, -0.70715638295, -0.710379447476, -0.713634742606, -0.714279355512, -0.718340416815], [-0.711765365224, -0.724560931444, -0.722369247503, -0.726784845983, -0.72494769918, -0.728621992799, -0.727880687945, -0.730072371842, -0.730169063782, -0.730845907354, -0.730104602467, -0.732618592899, -0.730749215401, -0.73229628649, -0.731135983188, -0.734230125256, -0.735744965582, -0.730781446088, -0.737066422059, -0.732747515477, -0.736228425243, -0.735197044577, -0.734326817112, -0.734584662293, -0.73342435903, -0.730555831519, -0.730684754112, -0.725270005612, -0.726108002436, -0.721885787838, -0.717824726532, -0.717147883005, -0.710476139452, -0.711249674934, -0.703578781432, -0.702676323345, -0.696004579975, -0.692813746133, -0.684240394829, -0.67934133696, -0.672121672803, -0.663354937875, -0.655812967451, -0.650043682499, -0.638440651315, -0.632123445558, -0.622744328924, -0.611689219083, -0.607595927736, -0.593865674939, -0.589933536879, -0.575333057211, -0.567501011901, -0.558411971797, -0.547131248426, -0.538364514917, -0.530081241095, -0.517382370075, -0.51100070404, -0.498624139668, -0.492371396341, -0.485183964551, -0.476449462421, -0.473194168256, -0.465555507761, -0.464234051759, -0.457014389609, -0.457755694206, -0.454371477587, -0.456530930071, -0.456982158954, -0.458819305118, -0.462396905535, -0.46897195505, -0.47374208902, -0.483926969825, -0.492210243146, -0.508003254901, -0.522893809026, -0.535270373741, -0.558895431386, -0.574559521866, -0.601278722161, -0.624001323916, -0.650913909799, -0.679824796629, -0.710411678102, -0.740547331832, -0.775582045369, -0.808135000648, -0.848326621873, -0.884908412339, -0.925744651385, -0.968127964584, -1.008577441074, -1.056762279125, -1.097276222847, -1.147588292081, -1.191615385176, -1.241476233341, -1.284697567014, -1.33227004555, -1.378778915937, -1.420968878904, -1.465318301289, -1.510505725619, -1.547055328546, -1.589825458321, -1.625085839421, -1.659056995213, -1.6933182298, -1.717781332923, -1.748690578516, -1.765740622068, -1.785755891413, -1.798164714248, -1.806254622338, -1.809703308258, -1.809252078319, -1.799163866215, -1.788269886665, -1.76541831494, -1.743694819196, -1.711302961563, -1.672851734771, -1.630113828191, -1.577964562881, -1.525267381534, -1.456487093395, -1.391864572571, -1.311513489345, -1.230872342166, -1.140529775998, -1.045288163425, -0.943826049219, -0.836916971325, -0.721821326526, -0.606467855284, -0.479189066374, -0.355326744083, -0.223052245422, -0.083783719617, 0.049554354938, 0.196719348996, 0.334666373306, 0.48295941228, 0.627545921343, 0.774259643201, 0.919458521707, 1.065463162938, 1.206891058243, 1.34793218853, 1.481882589672, 1.615349537597, 1.739276232442, 1.860205488455, 1.972754793568, 2.073636624006, 2.174131695086, 2.255288400978, 2.334833581771, 2.396265156012, 2.453506752411, 2.495084265497, 2.524027372682, 2.541045146617, 2.543430213434, 2.529861117134, 2.506655062122, 2.462015638659, 2.408770639614, 2.335897192413, 2.24555475284, 2.146123286002, 2.021197409573, 1.891179107926, 1.737793624341, 1.575093507418, 1.394763259411, 1.202088698055, 0.994652523619, 0.776225710175, 0.544100877349, 0.304208444897, 0.047813901563, -0.211159144441, -0.483798047303, -0.7653326994, -1.052572293041, -1.351124992534, -1.647808481302, -1.959221597519, -2.263576411537, -2.577342854314, -2.887370806551, -3.196786672335, -3.502560771377, -3.804693114694, -4.097801143999, -4.386429416404, -4.661940020556, -4.932841925659, -5.185952608819, -5.425397603927, -5.655914855497, -5.862258976218, -6.060545516593, -6.229662966251, -6.387080614154, -6.520099284844, -6.631684206844, -6.718579969795, -6.784170830334, -6.823106351241, -6.840704694108, -6.828811308327, -6.796128675609, -6.733793179361, -6.64683294574, -6.537890983214, -6.395138442166, -6.238010868241, -6.046911698304, -5.838214491566, -5.598736752886, -5.34024295002, -5.058736491301, -4.756151316888, -4.432584187887, -4.093063195321, -3.731174427893, -3.358005356716, -2.96743213227, -2.568350468634, -2.160405808323, -1.73857013707, -1.318604238285, -0.881105195248, -0.447989812003, -0.002143557587, 0.439770395346, 0.884520545481, 1.326466604942, 1.764770645786, 2.195178290564, 2.620235815048, 3.02843692896, 3.430288857773, 3.814124125672, 4.179072505695, 4.52316791251, 4.853211018603, 5.164689498048, 5.44345397781, 5.704814050875, 5.9364897071, 6.144959296661, 6.322745187771, 6.475552201279, 6.596772938093, 6.691693235321, 6.755704025392, 6.790030060846, 6.791222608696, 6.766114644038, 6.710580606664, 6.62197757689, 6.508234414488, 6.359295095206, 6.193789165152, 5.98938063049, 5.765923803883, 5.515522164724, 5.241753395342, 4.94510100651, 4.628981503492, 4.290397456829, 3.93847018769, 3.564207334467, 3.179985482758, 2.78126008812, 2.368385663559, 1.953803191747, 1.525587293446, 1.098338380085, 0.665416884865, 0.236459696272, -0.197138822371, -0.624291399669, -1.052507831657, -1.472989204735, -1.890312321264, -2.296774081073, -2.696242198286, -3.081722610934, -3.457050786674, -3.813749999477, -4.153560682818, -4.479544743602, -4.778809735956, -5.065569480639, -5.322515831455, -5.562960158558, -5.776523965273, -5.966945991103, -6.133227000213, -6.275431391187, -6.390561595666, -6.484773744206, -6.547657079024, -6.589880141444, -6.607413996422, -6.599259464388, -6.570734721027, -6.512073682302, -6.438199480229, -6.338024566655, -6.220122507215, -6.078304936196, -5.921564420508, -5.743229139087, -5.550132156053, -5.341113190445, -5.117300374375, -4.880176376789, -4.633899033522, -4.373504792794, -4.106825808411, -3.833475315589, -3.551261620261, -3.269950678431, -2.976327836394, -2.691053042014, -2.398881106403, -2.110996091378, -1.823433590916, -1.540995958539, -1.262200556184, -0.990302657263, -0.720725484573, -0.461558909037, -0.206614626238, 0.037919101747, 0.272267907717, 0.499590406638, 0.709766199878, 0.914688392123, 1.100852367279, 1.279925610207, 1.440724104466, 1.590016279132, 1.724740227003, 1.845605020756, 1.949516519928, 2.042534077976, 2.117470265228, 2.181157970384, 2.227731218564, 2.261766756197, 2.283038967805, 2.28664879767, 2.282748892171, 2.259220536969, 2.232630273161, 2.185960332916, 2.134133495452, 2.069672257958, 1.998023596367, 1.916286756241, 1.827588108294, 1.729381434927, 1.628402934234, 1.516723876331, 1.403529984368, 1.285275890746, 1.159995527641, 1.038131609861, 0.904245675988, 0.777353781392, 0.643338918953, 0.515641249901, 0.383495749512, 0.254637762314, 0.12616653192, 0.001015043127, -0.123491846328, -0.242132776215, -0.360709259352, -0.471582636471, -0.580715573951, -0.687463459203, -0.785315701171, -0.884682797774, -0.971737798179, -1.062015877006, -1.138015783997, -1.214273546373, -1.282054651605, -1.345678007751, -1.402500697588, -1.453940869169, -1.497774603487, -1.539384423977, -1.570196965704, -1.599140129151, -1.621701616217, -1.638977270006, -1.65506038846, -1.657896689984, -1.66540644294, -1.659475994245, -1.6561884629, -1.644843256998, -1.631628670883, -1.614481940201, -1.594917908013, -1.569326736977, -1.543928951467, -1.513599871748, -1.483303024612, -1.44929965047, -1.4141037433800001, -1.380390449999, -1.340682252615, -1.307678038826, -1.264521164743, -1.230131036731, -1.189617083625, -1.151584894783, -1.112360173922, -1.07342553161, -1.034780967818, -0.998328091321, -0.959328995068, -0.926228111175, -0.88954962641, -0.857383435016, -0.825056091908, -0.790665988836, -0.767621075384, -0.735583812304, -0.713473589391, -0.685658543145, -0.665159853888, -0.642662865403, -0.622808790165, -0.604050557231, -0.587870775927, -0.571852148146, -0.55921773777, -0.545165179484, -0.536269523486, -0.526535870989, -0.517736907139, -0.515287378725, -0.507165258283, -0.507906562927, -0.501395974404, -0.503748810838, -0.50236289347, -0.504393423551, -0.505682649001, -0.508293330553, -0.510388321916, -0.515867530145, -0.518059213454, -0.524569802165, -0.52875978496, -0.535786063969, -0.544327182925, -0.5475180161, -0.558959892661, -0.561989572689, -0.574462829917, -0.58013542245, -0.588805464462, -0.597636659824, -0.605597627963, -0.612591676972, -0.619392342204, -0.625580625296, -0.63495974198, -0.639891030191, -0.646466081183, -0.654330357939, -0.658165804432, -0.668737455312, -0.669672143973, -0.680662793387, -0.683982549693, -0.691427828421, -0.694360817091, -0.698679723403, -0.703030860409, -0.706511770053, -0.708606761965, -0.712861207147, -0.712990129697, -0.717695803943, -0.718082571675], [-0.71427935551, -0.722143632976, -0.72404524108, -0.724464239483, -0.726011310473, -0.728170763755, -0.726236924985, -0.730974829944, -0.729911218611, -0.734423509066, -0.732006210595, -0.73532596716, -0.734326817122, -0.73645403979, -0.734487970348, -0.737324267224, -0.735809426843, -0.737130883336, -0.735616042946, -0.735841657505, -0.735809426825, -0.734004510669, -0.735325967138, -0.73245743967, -0.733005360631, -0.72833191696, -0.728944299233, -0.724367547531, -0.724883237855, -0.721015560384, -0.718179263577, -0.713151282924, -0.711636442602, -0.704996929745, -0.70048463953, -0.69590788798, -0.690009680114, -0.685787465724, -0.676247195206, -0.67276628568, -0.662742555697, -0.659003801098, -0.648496611662, -0.643371939515, -0.635346509704, -0.629125995852, -0.617587426319, -0.609626458033, -0.598313503252, -0.590062459426, -0.5810056497, -0.569982771092, -0.560764808435, -0.550934463727, -0.54278011233, -0.530435778128, -0.525568951902, -0.515126225547, -0.509163557759, -0.49820514143, -0.491275554701, -0.483862508508, -0.476868460633, -0.470647948067, -0.466232351115, -0.461107680184, -0.458625921328, -0.455628472316, -0.453501250461, -0.455789625498, -0.455499549774, -0.462267983033, -0.463879514753, -0.471679328402, -0.477351920158, -0.487569031621, -0.495787843706, -0.511451932955, -0.524118573203, -0.541361964245, -0.557606205819, -0.579490809668, -0.601020877026, -0.62522608831, -0.651203985583, -0.68021156439, -0.710701753907, -0.739967180224, -0.77648450352, -0.809585379893, -0.849261310757, -0.886810020881, -0.928903255565, -0.969288268192, -1.013669885247, -1.056182127116, -1.102239745154, -1.14662137207, -1.194193838741, -1.239993622437, -1.283891800131, -1.333108043207, -1.377167381948, -1.425126637116, -1.467606680147, -1.512761873853, -1.55398492737, -1.595369137754, -1.630146058852, -1.665793211348, -1.697089221818, -1.725935700923, -1.7511078814, -1.771961148467, -1.789784729985, -1.802322475745, -1.811443766655, -1.812088380825, -1.814022223456, -1.80486870181, -1.794780489812, -1.772154532753, -1.749109577661, -1.716040874956, -1.677847493227, -1.632305515562, -1.582380167971, -1.52243108076, -1.459226701699, -1.386159741905, -1.308967265931, -1.22658566283, -1.13463156401, -1.040292410915, -0.936348537068, -0.829181615174, -0.712764515191, -0.595606129522, -0.467747190914, -0.342724567549, -0.20651793436, -0.070891470967, 0.071600097559, 0.213414807264, 0.359129407496, 0.506584448778, 0.654297325408, 0.800882123762, 0.94737022586, 1.096952464068, 1.236027525487, 1.379518182597, 1.512469436124, 1.645259542865, 1.769379623202, 1.890341111973, 2.001085504894, 2.107930002, 2.202365719158, 2.290387550084, 2.363937837082, 2.429043704874, 2.484931616791, 2.523350529433, 2.553260556559, 2.564992507132, 2.567732111023, 2.551584563608, 2.522383610465, 2.476454960925, 2.420470357663, 2.343825926324, 2.255417323432, 2.149281886744, 2.02712784304, 1.88930973233, 1.737761393734, 1.570162224343, 1.387124605696, 1.192451747079, 0.979407447398, 0.758434415577, 0.519895690267, 0.278069418051, 0.018709653029, -0.244840148886, -0.519219516403, -0.800979796488, -1.094955614997, -1.389286118006, -1.694833072763, -2.000702537671, -2.312986148011, -2.625850171815, -2.93652278559, -3.249355170025, -3.556031789992, -3.859840201111, -4.153141680389, -4.444058420266, -4.719923636027, -4.989923143988, -5.243775212777, -5.485573151627, -5.709837625206, -5.920081784168, -6.110826273553, -6.282651200402, -6.433461476219, -6.566415720895, -6.675067619843, -6.758450185193, -6.824588995507, -6.859173286962, -6.875772460093, -6.859624526589, -6.824137755937, -6.759191506871, -6.670909773554, -6.553490951991, -6.413091283668, -6.242394322554, -6.052036466714, -5.835281451458, -5.593354147693, -5.330863692688, -5.043555652639, -4.739294486152, -4.410602654685, -4.067600751817, -3.704519477413, -3.328385203867, -2.933009627492, -2.530962774319, -2.115669547686, -1.693124845495, -1.263489783148, -0.828827078002, -0.386300380611, 0.058256621803, 0.505617530523, 0.952494892089, 1.394537645167, 1.835839145116, 2.264699742945, 2.692754748947, 3.102277361797, 3.50377480462, 3.887610130214, 4.256039492337, 4.596750738449, 4.933014458055, 5.236660924787, 5.523160877875, 5.777881462885, 6.010846419604, 6.2183169114, 6.393878919235, 6.543752959125, 6.662072941399, 6.755220560184, 6.813171935692, 6.845145114857, 6.842824480732, 6.813043011561, 6.751642917357, 6.662395251416, 6.541206711077, 6.393330992815, 6.217124366535, 6.015197593409, 5.783360713855, 5.527576505504, 5.25171272113, 4.94664808477, 4.627563349858, 4.28085715874, 3.924030829939, 3.544707770738, 3.153072880645, 2.747514606141, 2.33567157803, 1.91096870489, 1.484364346433, 1.050250317358, 0.616329669921, 0.182570109135, -0.253639110055, -0.683982549674, -1.11674354445, -1.538546426072, -1.960156288454, -2.37003457972, -2.77282255144, -3.157593978725, -3.533856947913, -3.889943875657, -4.232300908653, -4.554030586337, -4.856518784492, -5.137799349038, -5.398001136619, -5.634513353977, -5.846497912768, -6.037081168104, -6.199268870824, -6.342891493272, -6.452542418278, -6.544337250969, -6.604609868697, -6.644834601269, -6.655342024898, -6.646123855617, -6.609670191078, -6.552620705694, -6.468625849124, -6.367838522832, -6.242458785089, -6.09641890151, -5.935520541452, -5.752995191112, -5.558125484081, -5.340597492477, -5.116043361895, -4.87360124189, -4.623746263204, -4.360483476925, -4.091000415003, -3.811332681458, -3.529409087399, -3.23955699438, -2.947416799028, -2.655115719545, -2.362782659945, -2.072834905165, -1.782017129298, -1.498902677582, -1.216852000067, -0.94714580684, -0.674474509818, -0.416436021814, -0.161008292115, 0.081430435869, 0.318454375505, 0.544294261008, 0.759046797099, 0.958908782521, 1.150551960331, 1.3256930704, 1.486878333803, 1.635815974349, 1.76644663758, 1.890308881358, 1.990932860833, 2.080437284391, 2.153504097989, 2.215451351557, 2.258769308244, 2.293352767506, 2.308662314137, 2.315462975972, 2.305793788522, 2.284328192747, 2.252226491756, 2.205878856903, 2.151119032095, 2.086722254951, 2.012656296172, 1.924892330287, 1.837353983908, 1.733055724553, 1.631819378809, 1.517948639422, 1.40256306617, 1.282407366842, 1.158480689198, 1.028752503791, 0.90166722756, 0.766975526221, 0.637891946316, 0.507035677319, 0.372086113208, 0.24358266189, 0.112178444411, -0.013037507026, -0.137544398039, -0.257474554668, -0.376889036173, -0.487536800959, -0.600956415756, -0.703159783003, -0.806040008442, -0.902216273391, -0.990496041248, -1.076519675291, -1.157612029636, -1.230034344694, -1.299201370965, -1.362437961015, -1.417391273061, -1.472054514814, -1.511633799747, -1.553630389705, -1.586860234387, -1.614417478835, -1.637397965769, -1.654061236775, -1.663472600955, -1.673560810025, -1.673045118824, -1.670337740007, -1.664310599148, -1.651837318588, -1.640621035564, -1.618220700996, -1.597947593358, -1.574483647939, -1.548860247294, -1.515694866593, -1.488202089125, -1.451394645029, -1.4187771924249999, -1.379552452264, -1.342003710407, -1.304745047244, -1.26558477698, -1.224361746464, -1.185652711274, -1.144719762673, -1.105301658294, -1.069815697357, -1.028044759736, -0.99458933488, -0.955622469533, -0.920974514364, -0.885778639949, -0.851807532229, -0.818900037683, -0.789795761301, -0.758145264994, -0.731458289609, -0.704674623302, -0.678825646667, -0.658520341464, -0.634411821073, -0.617297350552, -0.598152350062, -0.584067560455, -0.566953091032, -0.556284749658, -0.54139419487, -0.533626611202, -0.523312807272, -0.517317908815, -0.510646167026, -0.506133877904, -0.501943895193, -0.500235671484, -0.499494366853, -0.498591909034, -0.50139597438, -0.500976976118, -0.506456184285, -0.50623056982, -0.513804769405, -0.516931141161, -0.524021881292, -0.529114321967, -0.535786063895, -0.540975196562, -0.549806391361, -0.55557567561, -0.562118495244, -0.571110843455, -0.578523890504, -0.588128621042, -0.591673991433, -0.603309252486, -0.608208309861, -0.619456803495, -0.623614556202, -0.634895280692, -0.639504262485, -0.648754456759, -0.653363438624, -0.659712875235, -0.664805316804, -0.671477059967, -0.676956269335, -0.68040494819, -0.686593231814, -0.690654292999, -0.697777265362, -0.699163183093, -0.706028310381, -0.708445608764, -0.714053740998, -0.714376047447, -0.717309036158, -0.71921064424], [-0.710024910386, -0.716793345845, -0.719113952322, -0.719951949094, -0.719790795876, -0.722401478154, -0.721176713661, -0.722304786221, -0.722079171739, -0.725366697573, -0.723755165329, -0.727171613748, -0.725914618561, -0.729556681513, -0.729653373454, -0.733424359014, -0.730878137988, -0.732457439676, -0.733649973565, -0.732876438082, -0.73352105098, -0.731683904154, -0.733230975168, -0.731554981578, -0.731232675104, -0.729621142786, -0.729878987971, -0.727171613711, -0.728202994377, -0.722240324934, -0.722111402363, -0.716471039402, -0.713538050689, -0.709219144247, -0.704191163629, -0.700291255632, -0.695811196034, -0.689042760769, -0.681533020716, -0.677826496737, -0.670155603587, -0.663999550742, -0.655007201422, -0.648077613287, -0.636410120856, -0.629448302266, -0.617232889248, -0.61023884021, -0.598990346709, -0.591126070533, -0.580328806276, -0.569015851931, -0.560635885853, -0.550225389661, -0.54010496934, -0.529082091324, -0.5206376644, -0.509904862377, -0.501331513109, -0.490469788818, -0.485377348365, -0.475321390163, -0.471195868845, -0.464266282357, -0.459753993514, -0.455177243418, -0.45137402858, -0.450632723992, -0.448312118361, -0.44860219404, -0.449698035625, -0.454371477572, -0.456917697711, -0.464653049979, -0.471131407592, -0.483282357051, -0.492693702657, -0.508035485456, -0.522088043056, -0.539911585558, -0.558025204138, -0.578266045382, -0.601858873674, -0.626483083273, -0.654362588553, -0.681565251366, -0.71224882486, -0.744092702944, -0.780448873256, -0.816418277644, -0.855481826546, -0.892966075707, -0.936284075784, -0.975573246475, -1.019503634723, -1.062531567617, -1.107880111461, -1.154646808241, -1.200317665994, -1.247277754457, -1.292368467699, -1.34100455941, -1.386707663505, -1.432475233028, -1.474568508417, -1.519852625568, -1.559464144987, -1.598946744905, -1.634271588084, -1.669725356739, -1.700763521852, -1.729900077529, -1.753138415857, -1.775119757793, -1.792524340144, -1.80361170409, -1.81241068786, -1.814731299025, -1.812475149306, -1.804320779705, -1.791235111838, -1.769543845466, -1.745403046532, -1.71143188441, -1.674688884542, -1.627180834679, -1.577126564795, -1.518047706938, -1.453070640671, -1.38135737042, -1.30219882384, -1.218366841609, -1.127992046752, -1.030462059294, -0.926485956427, -0.819544650698, -0.701709403981, -0.584067560439, -0.458142461785, -0.329703393025, -0.19533390736, -0.059546292283, 0.082784121787, 0.226564897832, 0.371989421375, 0.519605614793, 0.666512725505, 0.816094969741, 0.962421918486, 1.109973628512, 1.251949444581, 1.393183959693, 1.527488899303, 1.660311237483, 1.784528010615, 1.906166343397, 2.016201663976, 2.121337939531, 2.217481880751, 2.303376491683, 2.379182923551, 2.442870644673, 2.496792488978, 2.535984937287, 2.564380125067, 2.57672445783, 2.578207067045, 2.561189292331, 2.532246183905, 2.485157231178, 2.427528865298, 2.350014206541, 2.259156075714, 2.150990109623, 2.029126141282, 1.8904055732, 1.734570563254, 1.566971394115, 1.382322245342, 1.184426326374, 0.970608492196, 0.747250395204, 0.509066205683, 0.264049101386, 0.004528180618, -0.260375311122, -0.538171131096, -0.820576031503, -1.115260933764, -1.414200435406, -1.71903833033, -2.028453192339, -2.340478978614, -2.655502488952, -2.968205671777, -3.281134781401, -3.587940359215, -3.891748806981, -4.186242869138, -4.475709255059, -4.752992675415, -5.02395915739, -5.276296406007, -5.519641480332, -5.744002687703, -5.952603092839, -6.14325092322, -6.315011419137, -6.465531641869, -6.595907403787, -6.7039791576, -6.785750168332, -6.847183205524, -6.8814774191, -6.895981552919, -6.878512129785, -6.840446842986, -6.77298653917, -6.683028767301, -6.562547959387, -6.417603667947, -6.247873640808, -6.051714154371, -5.832767417038, -5.588068236284, -5.322451369195, -5.03250039276, -4.723984745866, -4.39335907776, -4.046972951256, -3.68041076967, -3.302245985531, -2.904259747987, -2.499151006579, -2.082471893594, -1.657896690003, -1.226972430874, -0.788248690179, -0.34659224316, 0.101574571531, 0.549128852274, 0.99794004534, 1.440691873864, 1.883089223901, 2.315688590355, 2.742357703593, 3.153814185862, 3.556665354349, 3.938824725544, 4.307802055414, 4.648771194708, 4.982230886135, 5.286554247973, 5.568638621824, 5.826260029219, 6.055357318603, 6.260217140354, 6.435875871716, 6.582752456123, 6.700492300534, 6.79202838416, 6.848400448848, 6.877279453822, 6.870994402281, 6.840890618981, 6.775010405327, 6.682636322387, 6.559062678139, 6.407061384714, 6.228050656109, 6.020709080125, 5.788163116111, 5.529671511214, 5.249134254804, 4.943296081938, 4.619827965986, 4.270704476852, 3.909623703226, 3.527496586161, 3.134572481773, 2.724792004513, 2.311595300989, 1.885699903608, 1.453745269663, 1.018728785616, 0.581842919588, 0.146955279198, -0.290897715685, -0.723207244305, -1.155549266911, -1.581928938196, -2.002571919715, -2.413965101174, -2.817139893542, -3.202717146175, -3.57859340424, -3.93616301468, -4.277714337744, -4.599701926599, -4.90177118411, -5.183180734068, -5.440900782798, -5.678218832441, -5.889429891994, -6.078433861212, -6.241459615534, -6.379570719093, -6.490027451168, -6.577728923312, -6.635326350273, -6.672746961474, -6.681320504889, -6.670265146349, -6.631200736434, -6.571862818298, -6.486739855383, -6.380505427068, -6.254932292263, -6.10769984155, -5.942031249561, -5.758281107182, -5.558351102183, -5.339018167199, -5.109693837164, -4.865027781983, -4.613367876412, -4.346785311362, -4.07462709678, -3.794346993999, -3.510038333336, -3.217672254619, -2.925467618447, -2.630136865355, -2.335579904363, -2.043440480452, -1.75117234287, -1.467348834592, -1.185137020595, -0.912046622996, -0.642050483247, -0.38243270481, -0.12684383114, 0.114821354973, 0.354552660666, 0.579490085203, 0.792888933492, 0.993685605466, 1.181880108564, 1.358729441583, 1.517690794561, 1.66604828599, 1.79745248593, 1.91548099088, 2.016201663979, 2.103965635885, 2.175485381126, 2.236465717242, 2.279106831693, 2.310370537258, 2.325615622902, 2.329870065433, 2.319749649111, 2.297059289292, 2.261508911229, 2.215483582179, 2.159885760796, 2.090622159789, 2.014847978107, 1.928631081568, 1.837128369633, 1.73650439991, 1.632560682816, 1.518238714889, 1.402144068285, 1.277379392366, 1.154741939, 1.024562525132, 0.895253337089, 0.763333467718, 0.630382214794, 0.498140029227, 0.366220141981, 0.235944006455, 0.106634778363, -0.017582024409, -0.142443452805, -0.262051303755, -0.38333516252, -0.494305234496, -0.607112468088, -0.710218294224, -0.814581130586, -0.906986410225, -0.997683478167, -1.082933577324, -1.162446629846, -1.237157323255, -1.303036821458, -1.367562639148, -1.422934950654, -1.475503198335, -1.519562549385, -1.56052775785, -1.593177450511, -1.624086687772, -1.641459033707, -1.659766070563, -1.670950123395, -1.677976416022, -1.679749104576, -1.675945881909, -1.670273278632, -1.657606613718, -1.643715182568, -1.624344533351, -1.60468380868, -1.580091788639, -1.554403926346, -1.522463311488, -1.491167312477, -1.45545571143, -1.420968878936, -1.38248544425, -1.345903622526, -1.305615275514, -1.267679770787, -1.227520352303, -1.186426247372, -1.148136213419, -1.10778341951, -1.068171933565, -1.029688523456, -0.991205115721, -0.951239100204, -0.917203527712, -0.879010202787, -0.848133237989, -0.812679522248, -0.784026475241, -0.752343748533, -0.724947699177, -0.697519420203, -0.672411748598, -0.648980071258, -0.626805389693, -0.606790161664, -0.585743553728, -0.570885229008, -0.554640987151, -0.544262721671, -0.530758084501, -0.52411857322, -0.513837000056, -0.510388321919, -0.501105898678, -0.497657220622, -0.495175461647, -0.492758163962, -0.492790394595, -0.491340015991, -0.494530848929, -0.496110150111, -0.500461285963, -0.503974425287, -0.511032934651, -0.516125375253, -0.524537571479, -0.527309406293, -0.536205062214, -0.543360263805, -0.551353462011, -0.558379741184, -0.565631634866, -0.574204984823, -0.582230413998, -0.589450077279, -0.597894504944, -0.608272771146, -0.615846971723, -0.625032704438, -0.63031852964, -0.638956341598, -0.642888479894, -0.652074212929, -0.65616750453, -0.664354087814, -0.669253145555, -0.676279425834, -0.680243794981, -0.684788315789, -0.691041060696, -0.694844276739, -0.698196263731, -0.702128402385, -0.704610162007, -0.704384547489, -0.707962149067, -0.709509220038, -0.7142471249, -0.713699203924]]
  in  "Open":bool
  in  "Filter lf":bool caption="Scan"
  in  "Low cutoff freq: fl":dbl=40.0
  in  "Tab Control":T7(tab)
  out "Get data":bool
  out "Start Pos X":dbl
  out "Start Pos Y":dbl
  in  "Step X":dbl=1.0
  in  "Y - length":dbl=150.0
  in  "X - length":dbl=150.0
  in  "Step Y":dbl=1.0
  in  "Multiplier":dbl=10.0
  out "Cur. Pos Y":dbl=108.0 format="%#_4g"
  in  "Speed (mm/s)":dbl=6.0
  in  "Travel per Pulse (mm)":dbl=0.004
  in  "COM Y":refnum<visa-resource-name>="COM3"
  in  "COM X":refnum<visa-resource-name>="COM4"
  out "Completed":bool
  out "No. X":i32
  out "No. Y":i32
  in  "Baud Rate":u32=9600
  out "Cur. Pos X":dbl=88.516 format="%#_4g"
  in  "DAQ Pulser":bool=TRUE
  in  "No. Samples":dbl=500.0
  out "Sample per Channel AO":dbl=20000.0
  in  "Pulser Cycles":i32=10
  out "Actual Sample Rate":dbl=100000.0 format="%0.2f"
  in  "Physical Channel":tag="Dev3/ai1:2"
  in  "Min Voltage":dbl=-10.0
  in  "Max Voltage":dbl=10.0
  in  "Terminal Configuration":i32(ring)=10083 items=["default"=-1, "RSE"=10083, "NRSE"=10078, "Differential"=10106, "Pseudodifferential"=12529]
  in  "Sample Clock Source 2":tag="OnboardClock"
  in  "Sample Rate":dbl=100000.0
  out "Actual Sample Rate 2":dbl=400000.0 format="%0.2f"
  in  "Physical Channel(s)":tag="Dev3/ao0:1"
  in  "Min Voltage 2":dbl=-10.0
  in  "Max Voltage 2":dbl=10.0
  in  "Sample Clock Source":tag="OnboardClock"
  in  "Sample Rate 2":dbl=400000.0 format="%#_6p"
  # "Pulse Shape"
  # "Trigger Settings"
  # "Data Processing"
  # "Time gate = %T/2"
  # "3D Surface"
  # "Process"
  # "Repair line"
  # "Hall Sensors Signal"
  # "Feature Extraction"
  # "Power Spectal Density"
  # "COM Setting"
  # "Speed Setting"
  # "Scan Setting"
  # "Step > S*P/f"
  # "Pulser Channel"
  # "Pulser Timming"
  # "Sensor Channel"
  # "DAQ Timming"
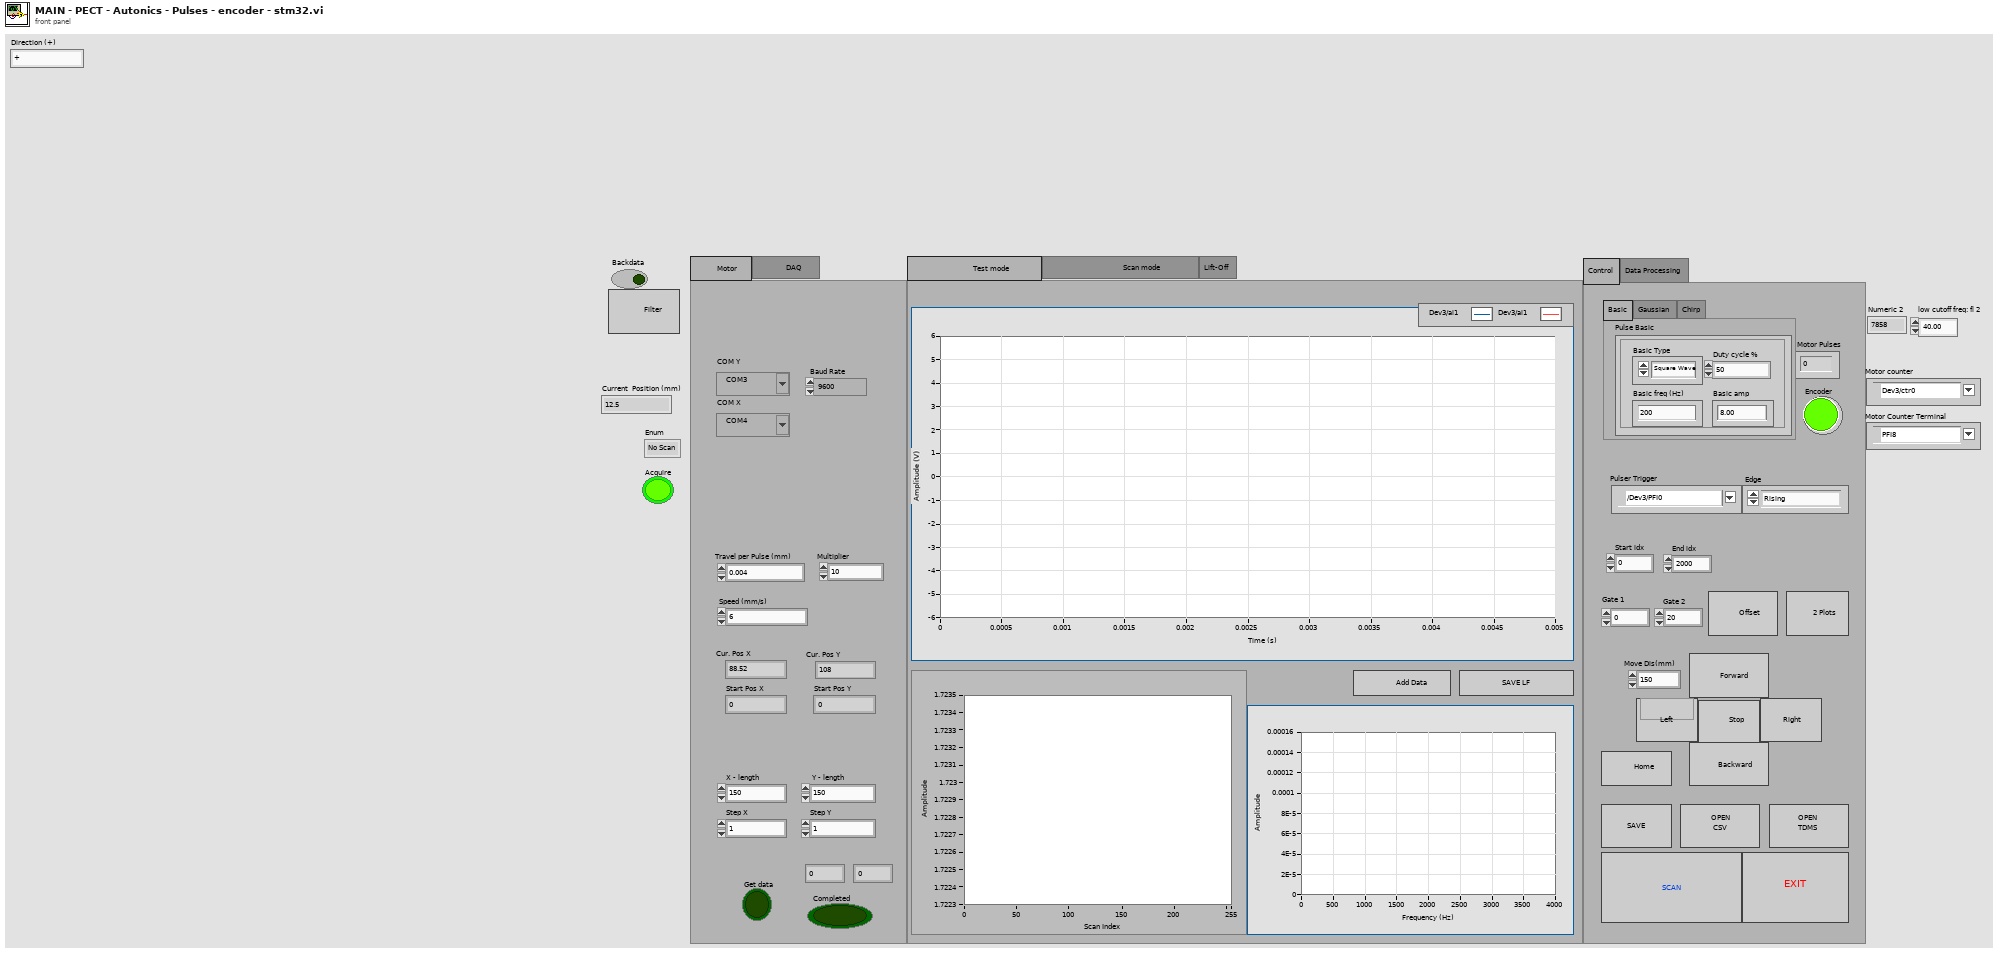
[diagram p1: front panel]
types:
  T1 = enum16{"No Scan", "Move X", "Wait X", "Move Y", "Wait Y"}
  T2 = typedef "Control 1.ctl" = dbl
  T3 = cluster{"Basic amp":T2, "Duty cycle %":dbl, "Basic freq (Hz)":u16, "Basic Type":u16}
  T4 = cluster{"Gauss amp":dbl, "Gauss Nor. Band":dbl, "Gauss atten (dB)":dbl, "Gauss freq (Hz)":dbl}
  T5 = cluster{"Chirp amp":dbl, "Chirp f2":dbl, "Chirp f1":dbl}
  T6 = enum32{"                    Test mode                   ", "                          Scan mode                      ", "Lift-Off"}
  T7 = enum32{"        Motor      ", "          DAQ        "}
  T8 = enum16{"open", "open or create", "create or replace", "create", "open (read-only)"}
  T9 = cluster{"Clients":refnum<k5>[], "Listener":refnum<k5>}
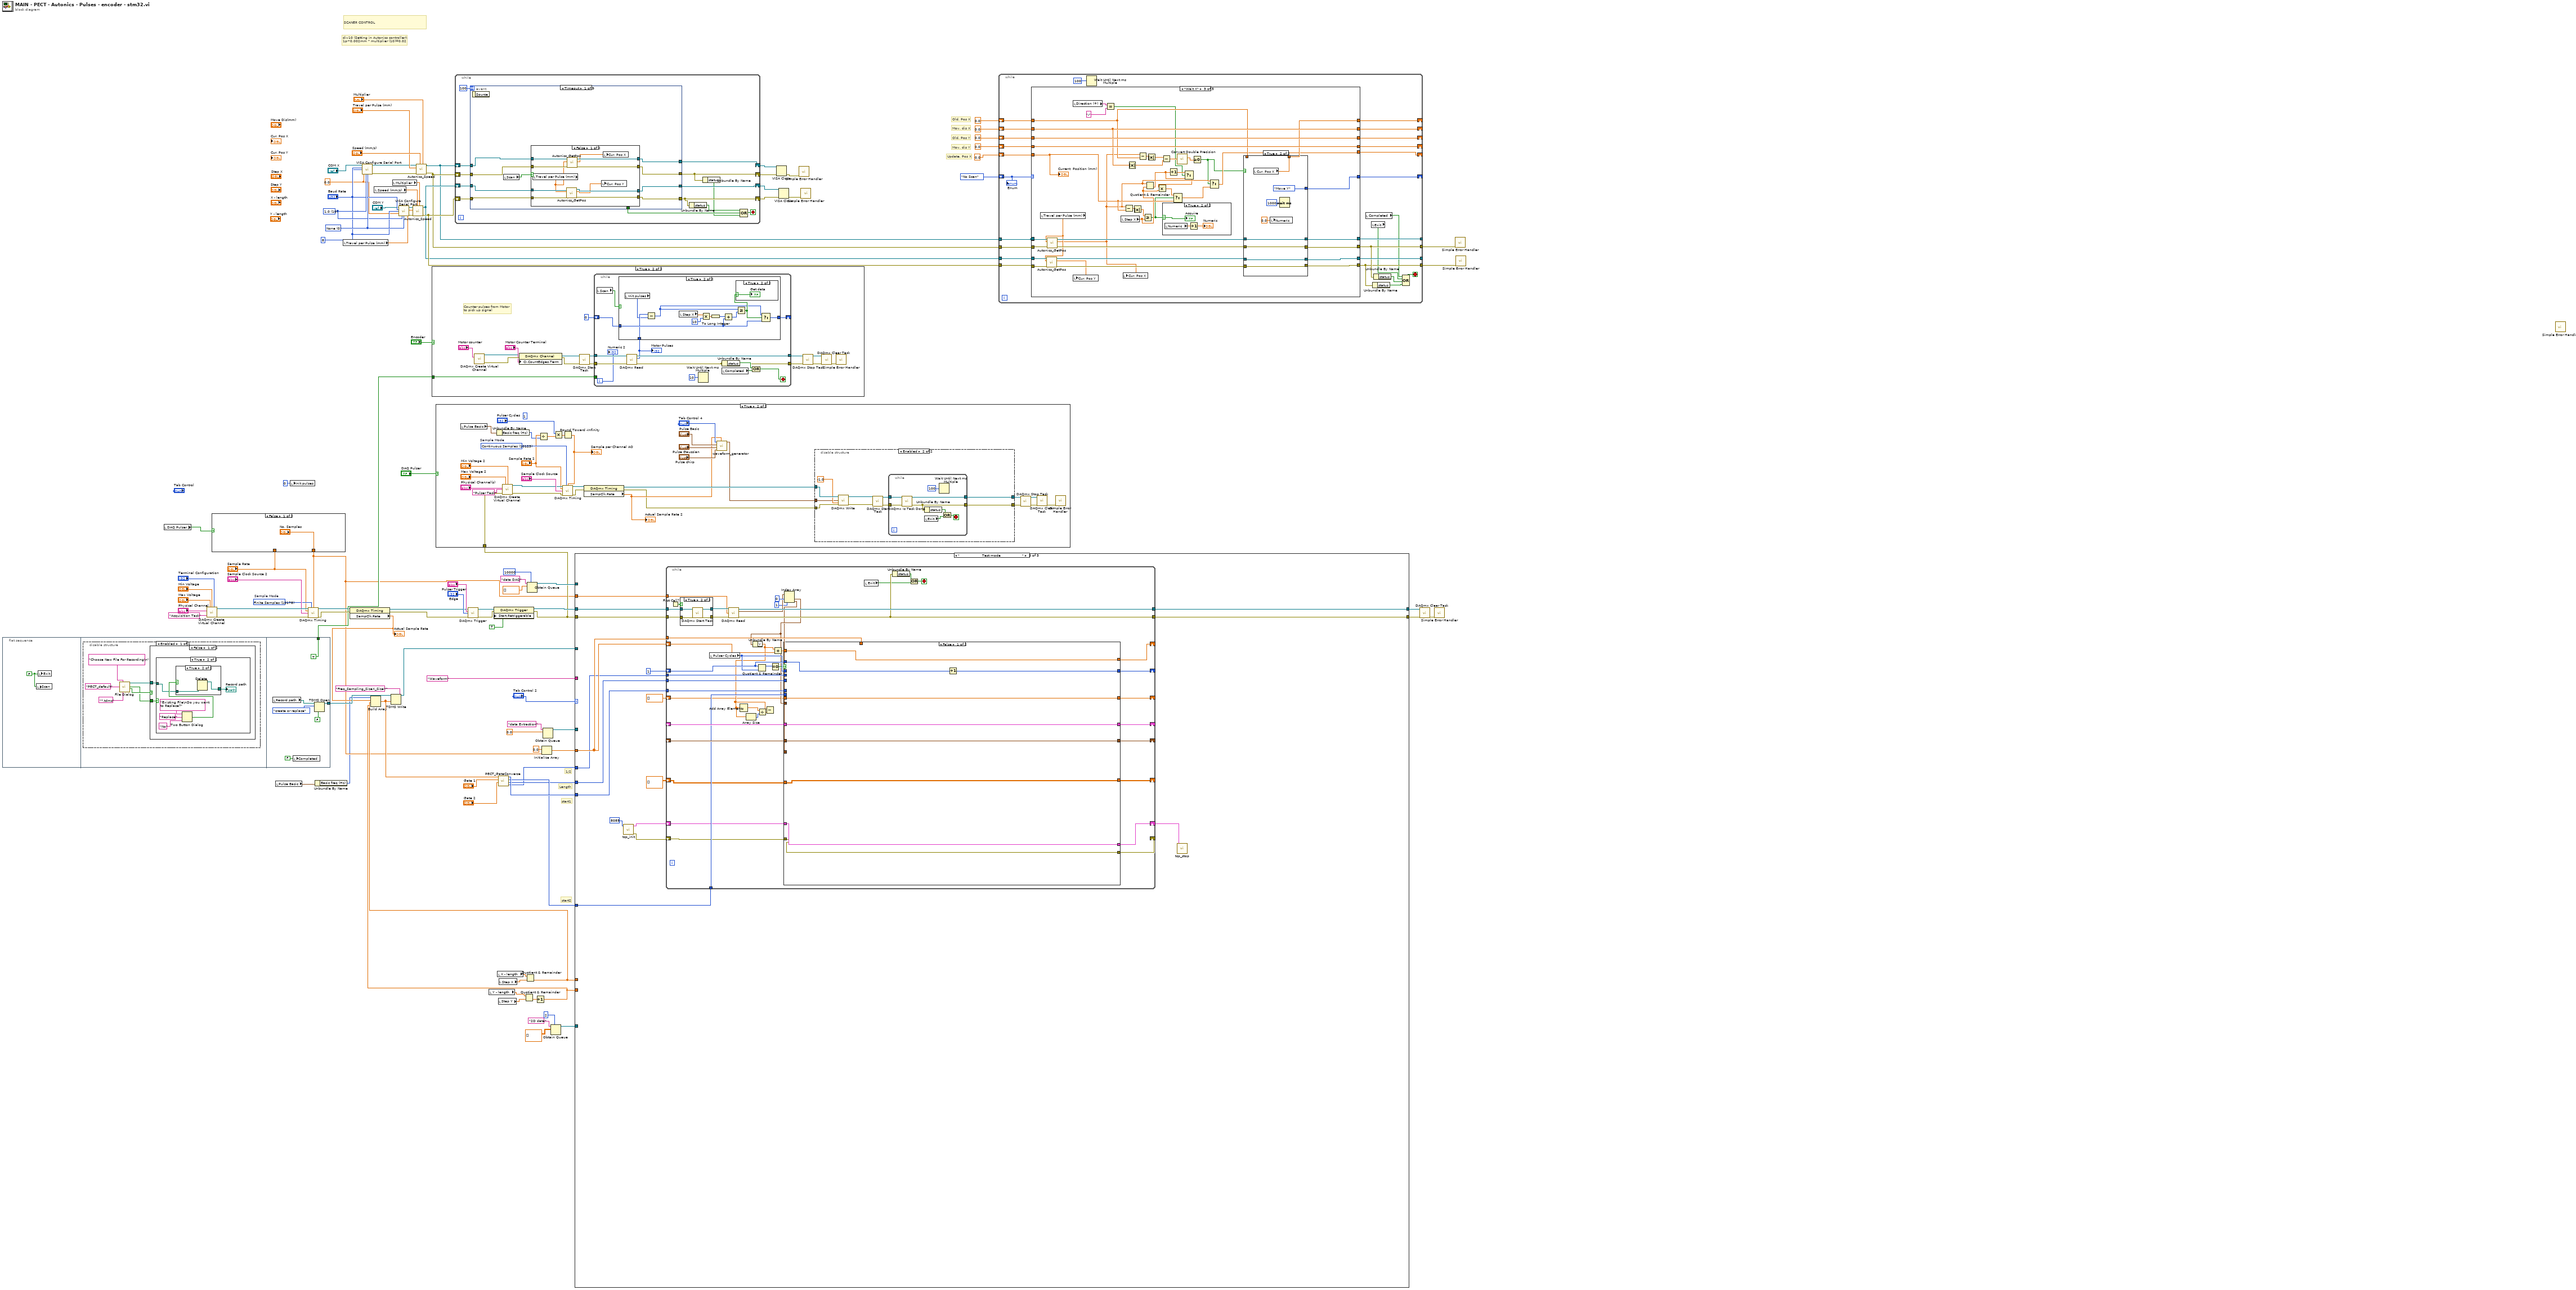
[diagram p0: block diagram]
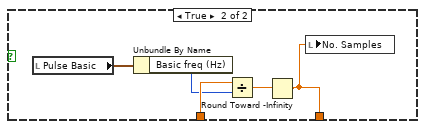
[diagram p5: hidden frame]
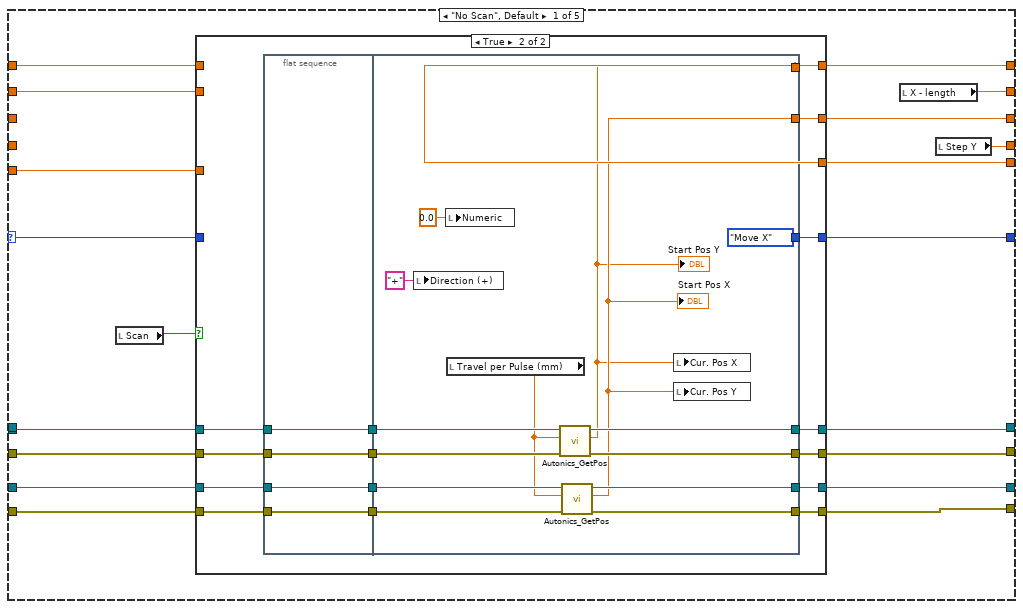
[diagram p6: hidden frame]
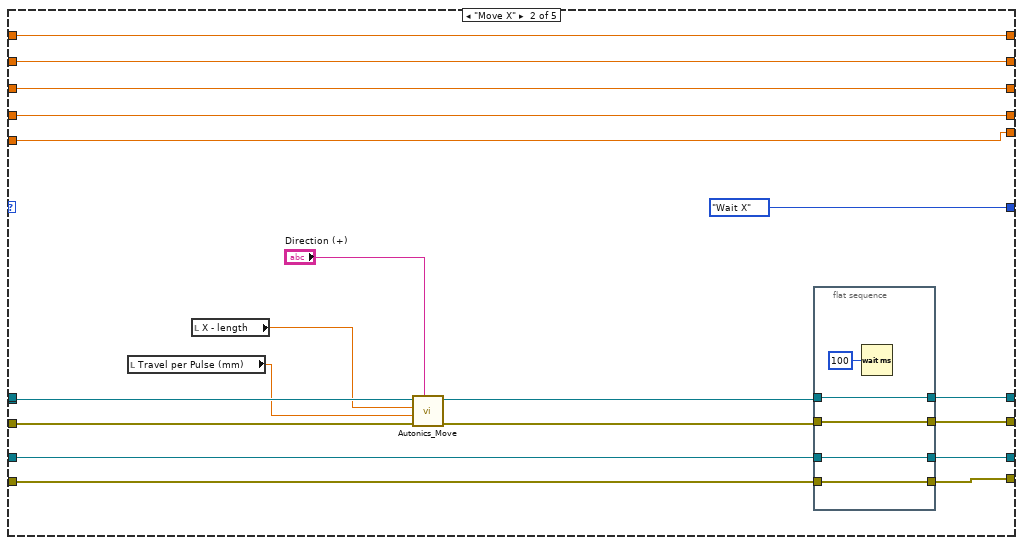
[diagram p8: hidden frame]
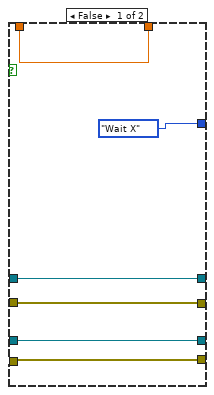
[diagram p10: hidden frame]
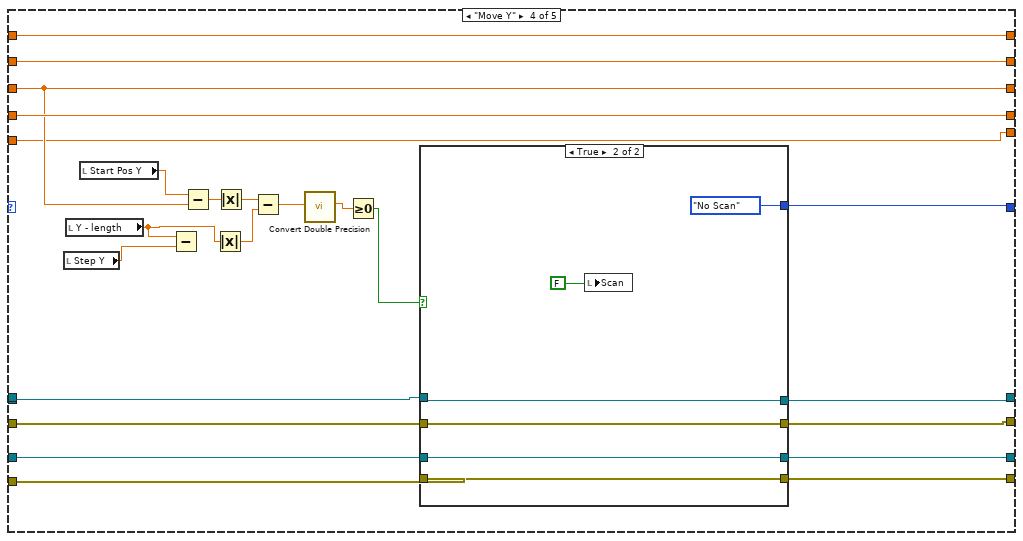
[diagram p11: hidden frame]
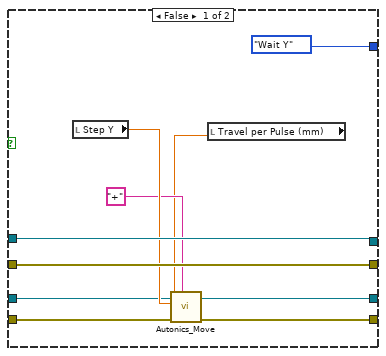
[diagram p12: hidden frame]
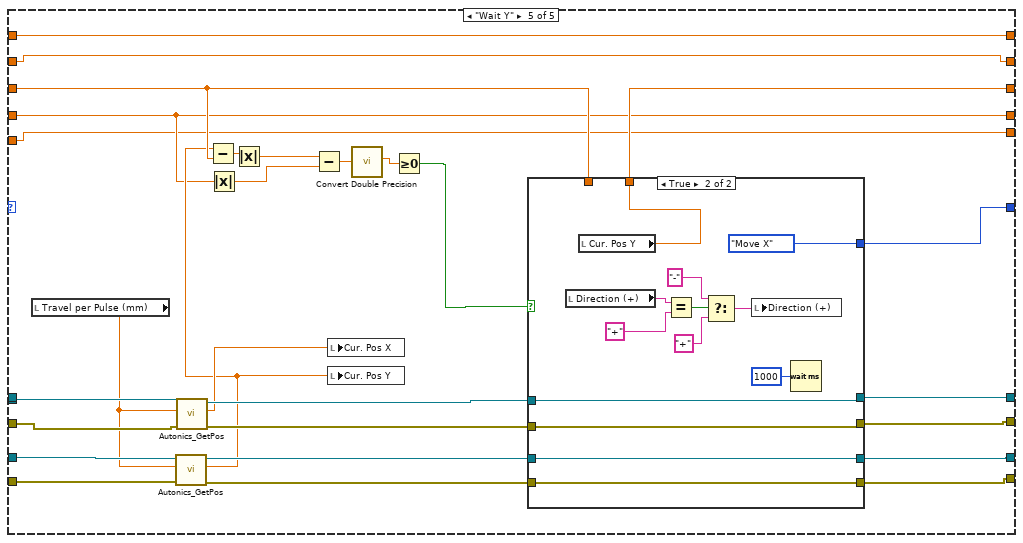
[diagram p13: hidden frame]
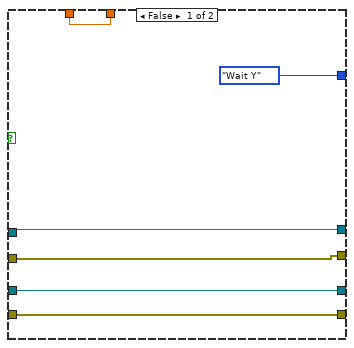
[diagram p14: hidden frame]
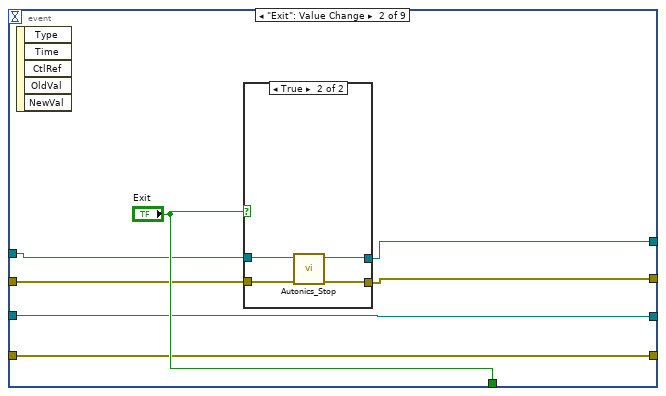
[diagram p16: hidden frame]
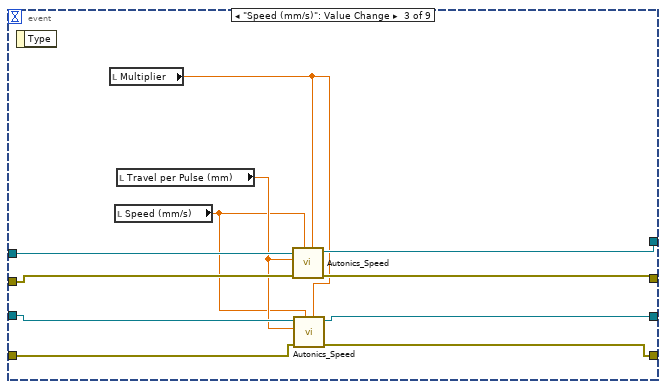
[diagram p18: hidden frame]
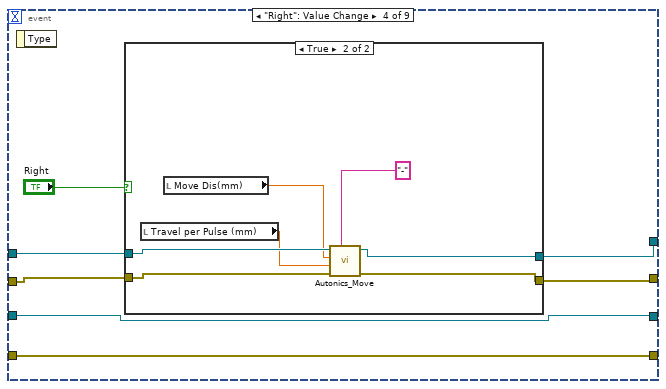
[diagram p19: hidden frame]
diagram:
  w22 = 0.0 ("Parity")
  w25 = u16 10 items=["1.0"=10, "1.5"=15, "2.0"=20] ("Stop bits")
  w26 = u16 0 items=["None", "XON/XOFF", "RTS/CTS", "XON/XOFF & RTS/CTS", "DTR/DSR", "XON/XOFF & DTR/DSR"] ("Flow control")
  w23 = u16 8 ("Data bits")
  w88 = 10178 items=["Finite Samples"=10178, "Continuous Samples"=10123, "Hardware Timed Single Point"=12522]  # Sample Mode
  # "Update. Pos X"
  # "Mov. dis Y"
  # "Old. Pos Y"
  # "Mov. dis X"
  # "Old. Pos X"
  # "div10 (Setting in Autonics controller):\n1p~0.002mm * multiplier (10)=0.02"
  # "SCANER CONTROL"
  # "1/2"
  # "start1"
  # "start2"
  # "Length"
  n1 = flat-sequence {
    tunnel: [w125] -> w68
    tunnel: [TRUE ("disable buffering (T)")] -> w50
    frame #0 {
      w101 = FALSE ("Exit")
      n2 = local write "Scan"(w101) -> ()
      n3 = local write "Exit"(w101) -> ()
    }
    frame #1 {
      n4 = disable-structure shown="Enabled" {
        frame Enabled {
          n5 = call "File Dialog"("prompt"="Choose New File For Recording\n" ("button label"), "default name"="PECT_default", "pattern (all files)"="*.tdms") -> ("selected path"=w107:path, "exists"=w103:bool, "cancelled"=w104:bool)  [unwired: 9 in, 1 out]
          n6 = case shown="False" w104 {
            tunnel: w107 -> [w108 _]
            tunnel: w103 -> [w109 _]
            frame False {
              n7 = case shown="True" w109 {
                tunnel: w108 -> [w110 w111]
                frame False {
                  n8 = local write "Record path"(w110) -> ()
                }
                frame True {
                  n9 = Two Button Dialog(message="Existing File\nDo you want to Replace?", 1:"No" ("F button name (\"Cancel\")"), 2:"Replace" ("T button name (\"OK\")")) -> (T button?=w112:bool)
                  n10 = case shown="True" w112 {
                    tunnel: w111 -> [_ w120]
                    tunnel: [path "" ("deleted path") w119] -> w113
                    frame False {
                      n11 = local write "Exit"(TRUE ("Exit")) -> ()
                    }
                    frame True {
                      n12 = Delete(path (use dialog)=w120) -> (deleted path=w119:path)  [unwired: 4 in, 2 out]
                    }
                  }
                  "Record path" <- w113
                }
              }
            }
            frame True {
              n13 = local write "Exit"(TRUE ("Exit")) -> ()
            }
          }
        }
        frame Disabled {
        }
      }
    }
    frame #2 {
      n14 = local read "Record path"() -> (w124:path)
      n15 = local write "Completed"(FALSE ("Completed")) -> ()
      n16 = TDMS Open(6:FALSE ("disable buffering (T)"), 10:T8."create or replace" ("operation"), 11:w124) -> (3:w125:refnum<k34>)  [unwired: 4 in, 1 out]
    }
  }
  n17 = local read "DAQ Pulser"() -> (w3:bool)
  n18 = call-poly <vilib>:"DAQmx Create Virtual Channel.vi"("maximum value"="Max Voltage", "minimum value"="Min Voltage", "input terminal configuration"="Terminal Configuration", "physical channels"="Physical Channel", "name to assign"="Acquisition Task") -> ("task out"=w98:refnum<k21>, "error out"=w99:errorcluster)  [unwired: 9 in]
  n19 = case shown="False" w3 {
    tunnel: ["No. Samples" w131] -> w7
    tunnel: "Sample Rate" -> [_ w132]
    frame False {
    }
    frame True {
      n20 = local read "Pulse Basic"() -> (w130:T3)
      n21 = Unbundle By Name(w130) -> ("Basic freq (Hz)"=w129:u16)
      n22 = Divide(x=w132, y=w129) -> (x/y=w133:dbl)
      n23 = Round Toward -Infinity(1:w133) -> (0:w131:dbl)
      n24 = local write "No. Samples"(w131) -> ()
    }
  }
  n25 = local read "Pulse Basic"() -> (w5:T3)
  n26 = local write "Init pulses"(0 ("Init pulses")) -> ()
  n27 = call-poly <vilib>:"DAQmx Timing.vi"("task/channels in"=w98, "sample mode"=w88, "samples per channel"=w7, "rate"="Sample Rate", "source"="Sample Clock Source 2", "error in"=w99) -> ("task out"=w48:refnum<k21>, "error out"=w100:errorcluster)  [unwired: 8 in]
  n28 = Unbundle By Name(w5) -> ("Basic freq (Hz)"=w4:u16)
  n29 = local read "Travel per Pulse (mm)"() -> (w21:dbl)
  n30 = property class="DAQmx Timing"(reference=w48, error in=w100) -> (reference out=w46:refnum<k21>, error out=w45:errorcluster, "SampClk.Rate"=w52:dbl)
  "Actual Sample Rate" <- w52
  n31 = call-poly "VISA Configure Serial Port"("VISA resource name"="COM X", "baud rate (9600)"="Baud Rate", "data bits (8)"=w23, "parity (0:none)"=w22, "stop bits (10: 1 bit)"=w25, "flow control (0:none)"=w26) -> ("VISA resource name out"=w11:refnum<visa-resource-name>, "error out"=w12:errorcluster)  [unwired: 8 in]
  n32 = local read "Speed (mm/s)"() -> (w19:dbl)
  n33 = local read "Multiplier"() -> (w20:dbl)
  n34 = call-poly "VISA Configure Serial Port"("VISA resource name"="COM Y", "baud rate (9600)"="Baud Rate", "data bits (8)"=w23, "parity (0:none)"=w22, "stop bits (10: 1 bit)"=w25, "flow control (0:none)"=w26) -> ("VISA resource name out"=w16:refnum<visa-resource-name>, "error out"=w17:errorcluster)  [unwired: 8 in]
  n35 = call "Autonics_Speed.vi"("Multiplier"=w20, "Speed (mm/s)"=w19, "error in (no error)"=w17, "Travel per  Pulse"=w21, "VISA resource name"=w16) -> ("error out"=w30:errorcluster, "VISA resource name out"=w29:refnum<visa-resource-name>)  [unwired: 5 in]
  n36 = call "Autonics_Speed.vi"("Multiplier"="Multiplier", "Speed (mm/s)"="Speed (mm/s)", "error in (no error)"=w12, "Travel per  Pulse"="Travel per Pulse (mm)", "VISA resource name"=w11) -> ("error out"=w28:errorcluster, "VISA resource name out"=w27:refnum<visa-resource-name>)  [unwired: 5 in]
  n37 = case shown="True" "Encoder" {
    tunnel: w50 -> [_ w148]
    frame False {
    }
    frame True {
      # "Counter pulses from Motor\nto pick up signal"
      n38 = call-poly <vilib>:"DAQmx Create Virtual Channel.vi"("counter"="Motor counter") -> ("task out"=w141:refnum<k21>, "error out"=w143:errorcluster)  [unwired: 13 in]
      n39 = property class="DAQmx Channel"(reference=w141, error in=w143, "CI.CountEdges.Term"="Motor Counter Terminal") -> (reference out=w136:refnum<k21>, error out=w137:errorcluster)
      n40 = call <vilib>:"DAQmx Start Task.vi"("task/channels in"=w136, "error in"=w137) -> ("task out"=w138:refnum<k21>, "error out"=w135:errorcluster)  [unwired: 12 in]
      n41 = while {
        tunnel: w138 -> [w162]
        tunnel: w135 -> [w161]
        tunnel: [w155] -> w145
        tunnel: [w160] -> w144
        tunnel: [w154] -> _
        tunnel: w148 -> [w154]
        shift-right: [w153] -> _
        shift-left: u32 0 ("data") -> [w152]
        i -> [w149]
        stop <- w156 stop-if-true
        n42 = local read "Scan"() -> (w150:bool)
        n43 = call-poly <vilib>:"DAQmx Read.vi"("task/channels in"=w162, "error in"=w161) -> ("task out"=w160:refnum<k21>, "data"=w151:u32, "error out"=w155:errorcluster)  [unwired: 11 in]
        "Motor Pulses" <- w151
        n44 = case shown="True" w150 {
          tunnel: [w163 w174] -> w153
          tunnel: w152 -> [w163 w173]
          tunnel: w151 -> [_ w166]
          frame False {
          }
          frame True {
            n45 = local read "Init pulses"() -> (w165:i32)
            n46 = Subtract(x=w166, y=w165) -> (x-y=w164:u32)
            n47 = local read "Step X"() -> (w172:dbl)
            n48 = Multiply(x=w172, y=10) -> (x*y=w170:dbl)
            n49 = To Long Integer(number=w170) -> (32bit integer=w169:i32)
            n50 = Add(x=w169, y=w173) -> (x+y=w168:u32)
            n51 = Greater Or Equal?(x=w164, y=w168) -> (x >= y?=w167:bool)
            n52 = case shown="True" w167 {
              selector: w167 -> [_ w175]
              frame False {
              }
              frame True {
                "Get data" <- w175
              }
            }
            n53 = Select(t=w164, s=w167, f=w173) -> (s? t:f=w174:u32)
          }
        }
        n54 = Wait Until Next ms Multiple(millisecond multiple=u32 10 ("milliseconds to wait")) -> ()  [unwired: 1 out]
        n55 = local read "Completed"() -> (w157:bool)
        n56 = Unbundle By Name(w155) -> ("status"=w158:bool)
        n57 = Compound Arithmetic op=OR(w158, w157) -> (w156:bool)
        "Numeric 2" <- w149
      }
      n58 = call <vilib>:"DAQmx Stop Task.vi"("task/channels in"=w144, "error in"=w145) -> ("task out"=w147:refnum<k21>, "error out"=w146:errorcluster)  [unwired: 12 in]
      n59 = call <vilib>:"DAQmx Clear Task.vi"("task in"=w147, "error in"=w146) -> ("error out"=w139:errorcluster)  [unwired: 13 in]
      n60 = call <vilib>:"Simple Error Handler.vi"("error in (no error)"=w139) -> ()  [unwired: 4 in, 5 out]
    }
  }
  n61 = while {
    shift-right: [w188] -> w41
    shift-left: w27 -> [w187]
    shift-right: [w178] -> w40
    shift-left: w28 -> [w186]
    shift-right: [w181] -> w42
    shift-left: w29 -> [w183]
    shift-right: [w180] -> w43
    shift-left: w30 -> [w182]
    stop <- w185 stop-if-true
    n62 = event shown="[0] Timeout" {
      selector: _ -> [_ _ _ _ _ _ _ _ _]
      dyn-events: _ -> [_ _ _ _ _ _ _ _ _]
      timeout: 100 -> [_ _ _ _ _ _ _ _ _]
      tunnel: w187 -> [w196 w218 w236 w241 w253 w273 w286 w309 w336]
      tunnel: w186 -> [w195 w217 w235 w240 w254 w272 w285 w308 w335]
      tunnel: [w192 w216 w234 w243 w253 w275 w286 w306 w338] -> w188
      tunnel: [w191 w215 w233 w242 w254 w274 w285 w305 w337] -> w178
      tunnel: [_ "Exit" _ _ _ _ _ _ _] -> w184
      tunnel: w183 -> [w194 w213 w232 w238 w258 w270 w289 w304 w333]
      tunnel: w182 -> [w193 w214 w229 w237 w257 w269 w290 w303 w331]
      tunnel: [w190 w213 w231 w238 w256 w270 w287 w301 w332] -> w181
      tunnel: [w189 w214 w230 w237 w255 w269 w288 w302 w330] -> w180
      event Timeout {
        n63 = event-data() -> ()  [unwired: 1 in, 1 out]
        n64 = local read "Scan"() -> (w197:bool)
        n65 = case shown="False" w197 {
          tunnel: w194 -> [w208 w210]
          tunnel: w193 -> [w207 w209]
          tunnel: [w206 w210] -> w190
          tunnel: [w205 w209] -> w189
          tunnel: w195 -> [w204 w211]
          tunnel: w196 -> [w203 w212]
          tunnel: [w202 w212] -> w192
          tunnel: [w201 w211] -> w191
          frame False {
            n66 = local read "Travel per Pulse (mm)"() -> (w200:dbl)
            n67 = call "Autonics_GetPos.vi"("error in (no error)"=w207, "Travel per Pulse (mm)"=w200, "VISA resource name"=w208) -> ("error out"=w205:errorcluster, "Current  Position (mm)"=w198:dbl, "VISA resource name out"=w206:refnum<visa-resource-name>)  [unwired: 6 in]
            n68 = call "Autonics_GetPos.vi"("error in (no error)"=w204, "Travel per Pulse (mm)"=w200, "VISA resource name"=w203) -> ("error out"=w201:errorcluster, "Current  Position (mm)"=w199:dbl, "VISA resource name out"=w202:refnum<visa-resource-name>)  [unwired: 6 in]
            n69 = local write "Cur. Pos Y"(w198) -> ()
            n70 = local write "Cur. Pos X"(w199) -> ()
          }
          frame True {
          }
        }
      }
      event "Exit": Value Change {
        n71 = event-data() -> ()  [unwired: 1 in, 5 out]
        n72 = case shown="True" "Exit" {
          tunnel: [w221 w224] -> w216
          tunnel: [w220 w225] -> w215
          tunnel: w218 -> [w221 w223]
          tunnel: w217 -> [w220 w222]
          frame False {
          }
          frame True {
            n73 = call "Autonics_Stop.vi"("error in (no error)"=w222, "VISA resource name"=w223) -> ("error out"=w225:errorcluster, "VISA resource name out"=w224:refnum<visa-resource-name>)  [unwired: 8 in]
          }
        }
      }
      event "Speed (mm/s)": Value Change {
        n74 = event-data() -> ()  [unwired: 1 in, 1 out]
        n75 = local read "Multiplier"() -> (w226:dbl)
        n76 = local read "Speed (mm/s)"() -> (w227:dbl)
        n77 = local read "Travel per Pulse (mm)"() -> (w228:dbl)
        n78 = call "Autonics_Speed.vi"("Multiplier"=w226, "Speed (mm/s)"=w227, "error in (no error)"=w235, "Travel per  Pulse"=w228, "VISA resource name"=w236) -> ("error out"=w233:errorcluster, "VISA resource name out"=w234:refnum<visa-resource-name>)  [unwired: 5 in]
        n79 = call "Autonics_Speed.vi"("Multiplier"=w226, "Speed (mm/s)"=w227, "error in (no error)"=w229, "Travel per  Pulse"=w228, "VISA resource name"=w232) -> ("error out"=w230:errorcluster, "VISA resource name out"=w231:refnum<visa-resource-name>)  [unwired: 5 in]
      }
      event "Right": Value Change {
        n80 = event-data() -> ()  [unwired: 1 in, 1 out]
        n81 = case shown="True" "Right" {
          tunnel: [w244 w250] -> w243
          tunnel: [w245 w246] -> w242
          tunnel: w241 -> [w244 w252]
          tunnel: w240 -> [w245 w251]
          frame False {
          }
          frame True {
            n82 = local read "Travel per Pulse (mm)"() -> (w248:dbl)
            n83 = local read "Move Dis(mm)"() -> (w249:dbl)
            n84 = call "Autonics_Move.vi"("Direction (+)"="-", "error in (no error)"=w251, "Travel per Pulse (mm)"=w248, "Move Distance (mm)"=w249, "VISA resource name"=w252) -> ("error out"=w246:errorcluster, "VISA resource name out"=w250:refnum<visa-resource-name>)  [unwired: 5 in]
          }
        }
      }
      event "Forward": Value Change {
        n85 = event-data() -> ()  [unwired: 1 in, 1 out]
        n86 = case shown="True" "Forward" {
          tunnel: [w260 w266] -> w256
          tunnel: [w261 w265] -> w255
          tunnel: w258 -> [w260 w268]
          tunnel: w257 -> [w261 w267]
          frame False {
          }
          frame True {
            n87 = local read "Travel per Pulse (mm)"() -> (w263:dbl)
            n88 = local read "Move Dis(mm)"() -> (w264:dbl)
            n89 = call "Autonics_Move.vi"("Direction (+)"="+", "error in (no error)"=w267, "Travel per Pulse (mm)"=w263, "Move Distance (mm)"=w264, "VISA resource name"=w268) -> ("error out"=w265:errorcluster, "VISA resource name out"=w266:refnum<visa-resource-name>)  [unwired: 5 in]
          }
        }
      }
      event "Left": Value Change {
        n90 = event-data() -> ()  [unwired: 1 in, 1 out]
        n91 = case shown="True" "Left" {
          tunnel: [w277 w282] -> w275
          tunnel: [w276 w281] -> w274
          tunnel: w273 -> [w277 w284]
          tunnel: w272 -> [w276 w283]
          frame False {
          }
          frame True {
            # "Moving distance"
            n92 = local read "Travel per Pulse (mm)"() -> (w278:dbl)
            n93 = local read "Move Dis(mm)"() -> (w279:dbl)
            n94 = call "Autonics_Move.vi"("Direction (+)"="+", "error in (no error)"=w283, "Travel per Pulse (mm)"=w278, "Move Distance (mm)"=w279, "VISA resource name"=w284) -> ("error out"=w281:errorcluster, "VISA resource name out"=w282:refnum<visa-resource-name>)  [unwired: 5 in]
          }
        }
      }
      event "Backward": Value Change {
        n95 = event-data() -> ()  [unwired: 1 in, 1 out]
        n96 = case shown="True" "Backward" {
          tunnel: [w293 w298] -> w287
          tunnel: [w292 w297] -> w288
          tunnel: w289 -> [w293 w300]
          tunnel: w290 -> [w292 w299]
          frame False {
          }
          frame True {
            # "Moving distance"
            n97 = local read "Travel per Pulse (mm)"() -> (w294:dbl)
            n98 = local read "Move Dis(mm)"() -> (w295:dbl)
            n99 = call "Autonics_Move.vi"("Direction (+)"="-", "error in (no error)"=w299, "Travel per Pulse (mm)"=w294, "Move Distance (mm)"=w295, "VISA resource name"=w300) -> ("error out"=w297:errorcluster, "VISA resource name out"=w298:refnum<visa-resource-name>)  [unwired: 5 in]
          }
        }
      }
      event "Home": Value Change {
        n100 = event-data() -> ()  [unwired: 1 in, 1 out]
        n101 = case shown="True" "Home" {
          tunnel: [w313 w325] -> w306
          tunnel: [w312 w324] -> w305
          tunnel: w309 -> [w313 w329]
          tunnel: w308 -> [w312 w328]
          tunnel: w304 -> [w311 w321]
          tunnel: w303 -> [w310 w320]
          tunnel: [w311 w319] -> w301
          tunnel: [w310 w318] -> w302
          frame False {
          }
          frame True {
            n102 = call "Autonics_Home.vi"("error in (no error)"=w328, "VISA resource name"=w329) -> ("error out"=w326:errorcluster, "VISA resource name out"=w327:refnum<visa-resource-name>)  [unwired: 8 in]
            n103 = call "Autonics_Home.vi"("error in (no error)"=w320, "VISA resource name"=w321) -> ("error out"=w323:errorcluster, "VISA resource name out"=w322:refnum<visa-resource-name>)  [unwired: 8 in]
            n104 = local read "Speed (mm/s)"() -> (w316:dbl)
            n105 = local read "Travel per Pulse (mm)"() -> (w317:dbl)
            n106 = local read "Multiplier"() -> (w315:dbl)
            n107 = local write "Home"(FALSE ("Home")) -> ()
            n108 = call "Autonics_Speed.vi"("Multiplier"=w315, "Speed (mm/s)"=w316, "error in (no error)"=w326, "Travel per  Pulse"=w317, "VISA resource name"=w327) -> ("error out"=w324:errorcluster, "VISA resource name out"=w325:refnum<visa-resource-name>)  [unwired: 5 in]
            n109 = call "Autonics_Speed.vi"("Multiplier"=w315, "Speed (mm/s)"=w316, "error in (no error)"=w323, "Travel per  Pulse"=w317, "VISA resource name"=w322) -> ("error out"=w318:errorcluster, "VISA resource name out"=w319:refnum<visa-resource-name>)  [unwired: 5 in]
          }
        }
      }
      event "Stop": Value Change {
        n110 = event-data() -> ()  [unwired: 1 in, 1 out]
        n111 = case shown="False" "Stop" {
          tunnel: [w340 w347] -> w338
          tunnel: [w342 w350] -> w337
          tunnel: w336 -> [w340 w349]
          tunnel: w335 -> [w342 w348]
          tunnel: w333 -> [w341 w346]
          tunnel: [w341 w345] -> w332
          tunnel: w331 -> [w339 w344]
          tunnel: [w339 w343] -> w330
          frame False {
          }
          frame True {
            n112 = call "Autonics_Stop.vi"("error in (no error)"=w348, "VISA resource name"=w349) -> ("error out"=w350:errorcluster, "VISA resource name out"=w347:refnum<visa-resource-name>)  [unwired: 8 in]
            n113 = call "Autonics_Stop.vi"("error in (no error)"=w344, "VISA resource name"=w346) -> ("error out"=w343:errorcluster, "VISA resource name out"=w345:refnum<visa-resource-name>)  [unwired: 8 in]
          }
        }
      }
    }
    n114 = Unbundle By Name(w180) -> ("status"=w179:bool)
    n115 = Unbundle By Name(w178) -> ("status"=w177:bool)
    n116 = Compound Arithmetic op=OR(w179, w184, w177) -> (w185:bool)
  }
  n117 = call-poly <vilib>:"DAQmx Trigger.vi"("task/channels in"=w46, "source"="Pulser Trigger", "edge"="Edge", "error in"=w45) -> ("task out"=w85:refnum<k21>, "error out"=w84:errorcluster)  [unwired: 10 in]
  n118 = local read "Y - length"() -> (w9:dbl)
  n119 = property class="DAQmx Trigger"(reference=w85, error in=w84, "Start.Retriggerable"=TRUE) -> (reference out=w70:refnum<k21>, error out=w51:errorcluster)
  n120 = case shown="True" "DAQ Pulser" {
    tunnel: w51 -> [_ w381]
    frame False {
    }
    frame True {
      (unwired) 1 ("x")
      w378 = 10123 items=["Finite Samples"=10178, "Continuous Samples"=10123, "Hardware Timed Single Point"=12522]  # Sample Mode
      n121 = local read "Pulse Basic"() -> (w352:T3)
      n122 = Unbundle By Name(w352) -> ("Basic freq (Hz)"=w351:u16)
      n123 = call-poly <vilib>:"DAQmx Create Virtual Channel.vi"("maximum value"="Max Voltage 2", "minimum value"="Min Voltage 2", "physical channels"="Physical Channel(s)", "name to assign"="Pulser Task", "error in"=w381) -> ("task out"=w372:refnum<k21>, "error out"=w371:errorcluster)  [unwired: 9 in]
      n124 = Divide(x="Sample Rate 2", y=w351) -> (x/y=w369:dbl)
      n125 = Multiply(x="Pulser Cycles", y=w369) -> (x*y=w368:dbl)
      n126 = Round Toward -Infinity(1:w368) -> (0:w360:dbl)
      "Sample per Channel AO" <- w360
      n127 = call-poly <vilib>:"DAQmx Timing.vi"("task/channels in"=w372, "sample mode"=w378, "samples per channel"=w360, "rate"="Sample Rate 2", "source"="Sample Clock Source", "error in"=w371) -> ("task out"=w380:refnum<k21>, "error out"=w379:errorcluster)  [unwired: 8 in]
      n128 = property class="DAQmx Timing"(reference=w380, error in=w379) -> (reference out=w367:refnum<k21>, error out=w353:errorcluster, "SampClk.Rate"=w355:dbl)
      "Actual Sample Rate 2" <- w355
      n129 = call "waveform_generator.vi"("Sampling rate"=w355, "Pulse chirp"="Pulse chirp", "Pulse Gaussian"="Pulse Gaussian", "Cluster Basic"="Pulse Basic", "Tab Control"="Tab Control 4") -> ("Waveform Graph"=w354:waveform(dbl)[])  [unwired: 6 in]
      n130 = disable-structure shown="Enabled" {
        disable-tunnel: w354 -> [w386 w407]
        disable-tunnel: [w385 w410] -> w364
        disable-tunnel: [w384 w409] -> w361
        disable-tunnel: w367 -> [w383 w411]
        disable-tunnel: w353 -> [w382 w406]
        frame Disabled {
          n131 = while {
            tunnel: w386 -> [w397]
            shift-right: [w393] -> w385
            shift-left: w383 -> [w391]
            shift-right: [w392] -> w384
            shift-left: w382 -> [w390]
            stop <- FALSE stop-if-true
            n132 = call-poly <vilib>:"DAQmx Write.vi"("task/channels in"=w391, "data"=w397, "timeout"=-1.0, "error in"=w390) -> ("task out"=w396:refnum<k21>, "error out"=w395:errorcluster)  [unwired: 9 in, 1 out]
            n133 = call <vilib>:"DAQmx Start Task.vi"("task/channels in"=w396, "error in"=w395) -> ("task out"=w389:refnum<k21>, "error out"=w388:errorcluster)  [unwired: 12 in]
            n134 = disable-structure shown="Enabled" {
              disable-tunnel: [w403 w405] -> w393
              disable-tunnel: [w402 w404] -> w392
              disable-tunnel: w389 -> [w401 w405]
              disable-tunnel: w388 -> [w400 w404]
              frame Disabled {
                n135 = call <vilib>:"DAQmx Wait Until Done.vi"("task/channels in"=w401, "error in"=w400) -> ("task out"=w399:refnum<k21>, "error out"=w398:errorcluster)  [unwired: 12 in]
                n136 = call <vilib>:"DAQmx Stop Task.vi"("task/channels in"=w399, "error in"=w398) -> ("task out"=w403:refnum<k21>, "error out"=w402:errorcluster)  [unwired: 12 in]
              }
              frame Enabled {
              }
            }
          }
        }
        frame Enabled {
          n137 = call-poly <vilib>:"DAQmx Write.vi"("task/channels in"=w411, "data"=w407, "timeout"=-1.0, "error in"=w406) -> ("task out"=w413:refnum<k21>, "error out"=w415:errorcluster)  [unwired: 9 in, 1 out]
          n138 = call <vilib>:"DAQmx Start Task.vi"("task/channels in"=w413, "error in"=w415) -> ("task out"=w412:refnum<k21>, "error out"=w414:errorcluster)  [unwired: 12 in]
          n139 = while {
            tunnel: w412 -> [w423]
            tunnel: w414 -> [w422]
            tunnel: [w420] -> w409
            tunnel: [w421] -> w410
            stop <- w417 stop-if-true
            n140 = call <vilib>:"DAQmx Is Task Done.vi"("task/channels in"=w423, "error in"=w422) -> ("task out"=w421:refnum<k21>, "error out"=w420:errorcluster)  [unwired: 11 in, 1 out]
            n141 = Unbundle By Name(w420) -> ("status"=w418:bool)
            n142 = local read "Exit"() -> (w416:bool)
            n143 = Wait Until Next ms Multiple(millisecond multiple=u32 100) -> ()  [unwired: 1 out]
            n144 = Compound Arithmetic op=OR(w418, w416) -> (w417:bool)
          }
        }
      }
      n145 = call <vilib>:"DAQmx Stop Task.vi"("task/channels in"=w364, "error in"=w361) -> ("task out"=w363:refnum<k21>, "error out"=w362:errorcluster)  [unwired: 12 in]
      n146 = call <vilib>:"DAQmx Clear Task.vi"("task in"=w363, "error in"=w362) -> ("error out"=w377:errorcluster)  [unwired: 13 in]
      n147 = call <vilib>:"Simple Error Handler.vi"("error in (no error)"=w377) -> ()  [unwired: 4 in, 5 out]
    }
  }
  n148 = local read "X - length"() -> (w75:dbl)
  n149 = local read "Step Y"() -> (w73:dbl)
  n150 = local read "Step X"() -> (w74:dbl)
  n151 = Quotient & Remainder(x=w9, y=w73) -> (floor(x/y)=w49:dbl)  [unwired: 1 out]
  n152 = Quotient & Remainder(x=w75, y=w74) -> (floor(x/y)=w66:dbl)  [unwired: 1 out]
  n153 = Obtain Queue(max queue size (-1, unlimited)=10000, name (unnamed)="data DAQ", element data type=dbl[] [] ("data")) -> (queue out=w80:refnum<queue>)  [unwired: 2 in, 2 out]
  n154 = Increment(x=w49) -> (x+1=w8:dbl)
  n155 = Build Array(w4, w52, w66, w8) -> (w57:dbl[])
  n156 = TDMS Write(0:w68, 5:"Freq_Sampling_SizeX_SizeY" ("group name in (Untitled)"), 9:w57) -> (4:w67:refnum<k34>)  [unwired: 3 in, 3 out]
  n157 = call "PECT_GateConverse.vi"("Gate 2"="Gate 2", "Gate 1"="Gate 1", "Freq_Sampling_SizeX_SizeY"=w57) -> ("Length T/2"=w58:i32, "Length"=w59:i32, "Start 2"=w60:i32, "Start 1"=w61:i32)  [unwired: 4 in, 1 out]
  n158 = Initialize Array(0.0 ("element"), w7) -> (w81:dbl[])
  n159 = Obtain Queue(name (unnamed)="data Extraction", element data type=0.0) -> (queue out=w78:refnum<queue>)  [unwired: 3 in, 2 out]
  n160 = Obtain Queue(max queue size (-1, unlimited)=2 ("최대 큐 크기(-1,제한없음)"), name (unnamed)="2D data", element data type=dbl[][] [] ("initialized array")) -> (queue out=w54:refnum<queue>)  [unwired: 2 in, 2 out]
  n161 = case shown="\"                    Test mode                   \"" "Tab Control 2" {
    tunnel: w70 -> [w458 w702 w733]
    tunnel: [w457 w702 w732] -> w91
    tunnel: [w456 w701 w731] -> w90
    tunnel: w81 -> [w453 _ w730]
    tunnel: w51 -> [w455 w701 w729]
    tunnel: w58 -> [w454 _ w728]
    tunnel: w80 -> [w452 _ _]
    tunnel: w78 -> [w432 _ _]
    tunnel: w66 -> [w428 _ _]
    tunnel: w8 -> [w429 _ _]
    tunnel: w59 -> [w440 _ w726]
    tunnel: w61 -> [w439 _ w725]
    tunnel: w60 -> [w438 _ w724]
    tunnel: w67 -> [w437 _ _]
    tunnel: "Waveform" ("group name in (Untitled)") -> [w434 _ _]
    tunnel: w54 -> [w430 _ _]
    tunnel: w7 -> [w425 _ w723]
    frame "                          Scan mode                      ", Default {
      # "Column"
      # "Row"
      n162 = Initialize Array(0.0 ("element"), w428, w429) -> (w445:dbl[][])
      n163 = local read "3D Surface"() -> (w441:refnum<k7>)
      n164 = Matrix Size(0:w445) -> (1:w446:i32, 2:w447:i32)
      n165 = Decrement(x=w446) -> (x-1=w450:i32)
      n166 = Decrement(x=w447) -> (x-1=w449:i32)
      n167 = call "Surface_AxesScale.vi"("Y-axis Max"=w449, "X-axis max"=w450, "3D Surface"=w441, "Auto Scale"=FALSE) -> ()  [unwired: 8 in]
      n168 = while {
        shift-right: [w504] -> _
        shift-left: 0 -> [w506]
        shift-right: [w503] -> _
        shift-left: 0 -> [w505]
        tunnel: w432 -> [w502]
        shift-right: [w494] -> w426
        shift-left: w445 -> [w501]
        shift-right: [w497] -> _
        shift-left: TRUE ("Output Direction") -> [w498]
        tunnel: w430 -> [w496]
        tunnel: [w495] -> w431
        stop <- w499 stop-if-true
        n169 = local read "Scan"() -> (w493:bool)
        n170 = local read "Completed"() -> (w492:bool)
        n171 = Compound Arithmetic op=AND(invert w493, invert w492) -> (w491:bool)
        n172 = case shown="False" w491 {
          tunnel: w506 -> [w523 w569]
          tunnel: w505 -> [w522 w568]
          tunnel: [w521 w569] -> w504
          tunnel: [w515 w568] -> w503
          tunnel: w502 -> [w520 w561]
          tunnel: w501 -> [w519 w565]
          tunnel: [w512 w548] -> w494
          tunnel: [w518 _] -> w490
          tunnel: w498 -> [w517 w567]
          tunnel: [w516 w567] -> w497
          tunnel: w496 -> [w513 w550]
          tunnel: [w511 w561] -> w495
          frame False {
            n173 = Dequeue Element(queue=w520, timeout in ms (-1)=5000) -> (queue out=w511:refnum<queue>, element=w514:dbl)  [unwired: 1 in, 2 out]
            n174 = call "EletoMatr_1channel.vi"("Input Array X"=w519, "Input data"=w514, "In Row"=w523, "In Column"=w522, "Input Direction"=w517) -> ("Completed"=w518:bool, "Out Array X"=w512:dbl[][], "Out Row"=w521:i32, "Output Direction"=w516:bool, "Out Column"=w515:i32)  [unwired: 6 in]
            n175 = Lossy Enqueue Element(queue=w513, element=w512) -> ()  [unwired: 1 in, 4 out]
          }
          frame True {
            n176 = local read "Gate 1"() -> (w564:dbl)
            n177 = local read "Gate 2"() -> (w563:dbl)
            n178 = Wait Until Next ms Multiple(millisecond multiple=u32 100 ("ms 배수")) -> ()  [unwired: 1 out]
            n179 = local read "Offset"() -> (w555:bool)
            n180 = call "TDMS_Open.vi"("Offset"=w555, "Gate 2"=w563, "Gate 1"=w564, "Input 2D"=w565, "Open"="Open tdms") -> ("Output 2D"=w528:dbl[][])  [unwired: 5 in, 1 out]
            n181 = case shown="True" "Open tdms" {
              tunnel: w528 -> [_ w570]
              frame False {
              }
              frame True {
                n182 = global write "Global_data.vi" "global 2d graph"(w570) -> ()
              }
            }
            n183 = call "RepairLine.vi"("Repair Line Col"="Repair Line Col", "Repair Line Row"="Repair Line Row", "Line Col"="Line Col", "Line Row"="Line Row", "Array In"=w528) -> ("Array Repaired"=w542:dbl[][])  [unwired: 6 in]
            n184 = call "CSV Open.vi"("2D Array In"=w542, "Open"="Open csv") -> ("2D Array Out"=w549:dbl[][])  [unwired: 9 in]
            n185 = call "Backdata.vi"("Backindex"="Backindex", "Array in"=w549, "Backdata"="Backdata") -> ("Array out"=w531:dbl[][])
            n186 = call "TrimXY.vi"("X-max"="Y-max", "X-min"="Y-min", "Y-max"="X-max", "Y-min"="X-min", "Array In"=w531, "Trim data"="Trim data") -> ("Array Trim Out"=w530:dbl[][])  [unwired: 5 in]
            n187 = global read "Global_data.vi" "global 2d graph"() -> (w525:dbl[][])
            n188 = call "Inverse.vi"(10:"Inverse"=w530, 11:"Inverse"="Inverse") -> ("Array out"=w526:dbl[][])  [unwired: 9 in]
            n189 = call "Return data.vi"("Array Return"=w525, "Array Input"=w526, "Return"="Return") -> ("Array out"=w524:dbl[][])  [unwired: 8 in]
            n190 = call "Abs.vi"("Input"=w524, "Abs"="Abs") -> ("Array out"=w554:dbl[][])  [unwired: 9 in]
            n191 = call "DiffX.vi"("Array in"=w554, "DiffX"="DiffX") -> ("Array out"=w559:dbl[][])  [unwired: 1 in]
            n192 = call "DiffY.vi"("Array in"=w559, "DiffY"="DiffY") -> ("Array out"=w557:dbl[][])  [unwired: 1 in]
            n193 = call "Odd.vi"("Odd"="Odd", "Array In"=w557) -> ("Array Out"=w546:dbl[][])  [unwired: 9 in]
            n194 = call "Filter_Lowpass - 2D.vi"("Filter"="Filter", "Input 2D"=w546, "low cutoff freq: fl"="low cutoff freq: fl") -> ("Output"=w545:dbl[][])  [unwired: 6 in]
            n195 = case shown="True" TRUE {
              tunnel: w545 -> [w571 w572]
              tunnel: [w571 w572] -> w548
              tunnel: w550 -> [_ w573]
              frame False {
              }
              frame True {
                n196 = local read "3D Surface"() -> (w577:refnum<k7>)
                n197 = Matrix Size(0:w572) -> (1:w578:i32, 2:w575:i32)
                n198 = Decrement(x=w578) -> (x-1=w576:i32)
                n199 = Decrement(x=w575) -> (x-1=w574:i32)
                n200 = call "Surface_AxesScale.vi"("Y-axis Max"=w574, "X-axis max"=w576, "3D Surface"=w577, "Auto Scale"=FALSE) -> ()  [unwired: 8 in]
                n201 = Lossy Enqueue Element(queue=w573, element=w572) -> ()  [unwired: 1 in, 4 out]
              }
            }
          }
        }
        "Output" <- w494
        n202 = case shown="True" w490 {
          selector: w490 -> [w507 w508]
          tunnel: [w507 w508] -> w489
          frame False {
          }
          frame True {
            n203 = Wait (ms)(milliseconds to wait=u32 200) -> ()  [unwired: 1 out]
          }
        }
        "Completed" <- w489
        n204 = local read "Exit"() -> (w500:bool)
        n205 = Compound Arithmetic op=OR(w489, w500) -> (w499:bool)
        "No. Y" <- w505
        "No. X" <- w506
      }
      n206 = while {
        tunnel: w458 -> [w589]
        tunnel: [w588] -> w457
        tunnel: [w587] -> w456
        tunnel: w455 -> [w586]
        tunnel: w452 -> [w585]
        tunnel: w425 -> [w580]
        stop <- w581 stop-if-true
        n207 = case shown="True" "Scan" {
          tunnel: w589 -> [w591 w597]
          tunnel: [w591 w596] -> w588
          tunnel: [w590 w595] -> w587
          tunnel: w586 -> [w590 w594]
          tunnel: w585 -> [_ w593]
          tunnel: w580 -> [_ w592]
          frame False {
          }
          frame True {
            n208 = while {
              tunnel: w597 -> [w611]
              tunnel: [w614] -> w596
              tunnel: [w613] -> w595
              tunnel: w594 -> [w610]
              tunnel: w593 -> [w612]
              tunnel: w592 -> [w602]
              stop <- w603 stop-if-true
              n209 = First Call?() -> (First Call?: T/F=w607:bool)
              n210 = case shown="True" w607 {
                tunnel: w611 -> [w615 w621]
                tunnel: w610 -> [w616 w620]
                tunnel: [w615 w619] -> w609
                tunnel: [w616 w618] -> w608
                frame False {
                }
                frame True {
                  n211 = local read "Motor Pulses"() -> (→"Init pulses":i32)
                  n212 = call <vilib>:"DAQmx Start Task.vi"("task/channels in"=w621, "error in"=w620) -> ("task out"=w619:refnum<k21>, "error out"=w618:errorcluster)  [unwired: 12 in]
                }
              }
              n213 = call-poly <vilib>:"DAQmx Read.vi"("task/channels in"=w609, "timeout"=w602, "error in"=w608) -> ("task out"=w614:refnum<k21>, "data"=w600:waveform(dbl)[], "error out"=w613:errorcluster)  [unwired: 10 in]
              n214 = Index Array(array=w600, index=0 ("index (row)")) -> (element=w599:waveform(dbl))
              n215 = Unbundle By Name(w599) -> ("Y"=w598:dbl[])
              n216 = Enqueue Element(queue=w612, element=w598) -> ()  [unwired: 2 in, 3 out]
              n217 = Unbundle By Name(w613) -> ("status"=w604:bool)
              n218 = local read "Completed"() -> (w606:bool)
              n219 = local read "Exit"() -> (w605:bool)
              n220 = Compound Arithmetic op=OR(w604, w606, w605) -> (w603:bool)
            }
          }
        }
        n221 = local read "Completed"() -> (w582:bool)
        n222 = local read "Exit"() -> (w583:bool)
        n223 = Compound Arithmetic op=OR(w582, w583) -> (w581:bool)
      }
      n224 = while {
        shift-right: [w636] -> _
        shift-left: w453 -> [w640]
        tunnel: w453 -> [w639]
        tunnel: w454 -> [w638]
        tunnel: w452 -> [w637]
        tunnel: w432 -> [w635]
        shift-right: [w632] -> _
        shift-left: 0 -> [w633]
        tunnel: w440 -> [w631]
        tunnel: w439 -> [w630]
        tunnel: w438 -> [w629]
        tunnel: w437 -> [w628]
        tunnel: [w627] -> w436
        tunnel: [w626] -> w435
        tunnel: w434 -> [w625]
        stop <- w622 stop-if-true
        n225 = local read "Scan"() -> (w634:bool)
        n226 = case shown="True" w634 {
          tunnel: w640 -> [w644 w655]
          tunnel: w639 -> [_ w661]
          tunnel: w638 -> [_ w660]
          tunnel: w637 -> [_ w659]
          tunnel: [w644 w658] -> w636
          tunnel: w635 -> [_ w657]
          tunnel: w633 -> [w643 w653]
          tunnel: [w643 w652] -> w632
          tunnel: w631 -> [_ w651]
          tunnel: w630 -> [_ w650]
          tunnel: w629 -> [_ w649]
          tunnel: w628 -> [w641 w648]
          tunnel: [w641 w647] -> w627
          tunnel: [_ w646] -> w626
          tunnel: w625 -> [_ w645]
          frame False {
            n227 = Wait Until Next ms Multiple(millisecond multiple=u32 100 ("ms 배수")) -> ()  [unwired: 1 out]
          }
          frame True {
            n228 = local read "Pulser Cycles"() -> (w654:i32)
            n229 = Increment(x=w653) -> (x+1=w652:i32)
            n230 = Dequeue Element(queue=w659) -> (element=w656:dbl[])  [unwired: 2 in, 3 out]
            n231 = Quotient & Remainder(x=w652, y=w654) -> (x-y*floor(x/y)=w662:i32)  [unwired: 1 out]
            n232 = Add(x=w656, y=w655) -> (x+y=w664:dbl[])
            n233 = Equal To 0?(x=w662) -> (x = 0?=w663:bool)
            n234 = case shown="True" w663 {
              tunnel: w654 -> [_ w689]
              tunnel: w664 -> [w666 w687]
              tunnel: [w666 w690] -> w658
              tunnel: w661 -> [_ w690]
              tunnel: w660 -> [_ w683]
              tunnel: w657 -> [_ w688]
              tunnel: w651 -> [_ w684]
              tunnel: w650 -> [_ w686]
              tunnel: w649 -> [_ w685]
              tunnel: w648 -> [w665 w681]
              tunnel: [w665 w679] -> w647
              tunnel: [_ w678] -> w646
              tunnel: w645 -> [_ w680]
              frame False {
                n235 = disable-structure shown="Enabled" {
                  frame Disabled {
                    n236 = Wait Until Next ms Multiple(millisecond multiple=u32 100 ("ms 배수")) -> ()  [unwired: 1 out]
                  }
                  frame Enabled {
                  }
                }
              }
              frame True {
                n237 = Divide(x=w687, y=w689) -> (x/y=w672:dbl[])
                n238 = local read "Start idx"() -> (w671:i32)
                n239 = local read "End idx"() -> (w676:i32)
                n240 = local read "Offset"() -> (w682:bool)
                n241 = Subtract(x=w676, y=w671) -> (x-y=w673:i32)
                n242 = call "PECT_Feature extraction.vi"("Length T/2"=w683, "Offset"=w682, "Length"=w684, "Start 2"=w685, "Start 1"=w686, "Pulse signal in"=w672) -> ("Feature extraction out"=w668:dbl)  [unwired: 5 in]
                n243 = Array Subset(array=w672, index=w671, length=w673) -> (w670:dbl[])
                n244 = Absolute Value(x=w670) -> (abs(x)=w669:dbl[])
                n245 = Array Size(array=w670) -> (size(s)=w674:i32)
                n246 = Add Array Elements(numeric array=w669) -> (sum=w675:dbl)
                n247 = local read "Get data"() -> (w677:bool)
                n248 = Divide(x=w675, y=w674) -> ()  [unwired: 1 out]
                n249 = case shown="True" w677 {
                  tunnel: w688 -> [_ w699]
                  tunnel: w668 -> [_ w698]
                  tunnel: w681 -> [w691 w697]
                  tunnel: w680 -> [_ w696]
                  tunnel: w672 -> [_ w692]
                  tunnel: [w691 w695] -> w679
                  tunnel: [_ w694] -> w678
                  frame False {
                  }
                  frame True {
                    n250 = TDMS Write(0:w697, 5:w696, 9:w692) -> (4:w695:refnum<k34>, 15:w694:errorcluster)  [unwired: 3 in, 2 out]
                    n251 = Enqueue Element(queue=w699, element=w698) -> ()  [unwired: 2 in, 3 out]
                    n252 = local write "Get data"(FALSE ("Acquire")) -> ()
                  }
                }
              }
            }
          }
        }
        n253 = local read "Completed"() -> (w624:bool)
        n254 = local read "Exit"() -> (w623:bool)
        n255 = Compound Arithmetic op=OR(w624, w623) -> (w622:bool)
        "No.data" <- w633
      }
      n256 = while {
        tunnel: w430 -> [w486]
        tunnel: w429 -> [_]
        tunnel: w428 -> [_]
        tunnel: [w483] -> w427
        stop <- w484 stop-if-true
        n257 = local read "Output"() -> (w474:dbl[][])
        n258 = local read "No. Y"() -> (w481:i32)
        n259 = call "CursorPosition.vi"("Cursor No."=1.0, "Cursor"="Cursor", "3D Surface Analysis"="3D Surface") -> ("Cursor Y"=w476:dbl)  [unwired: 6 in, 2 out]
        n260 = Dequeue Element(queue=w486, timeout in ms (-1)=3000) -> (queue out=w483:refnum<queue>)  [unwired: 1 in, 3 out]
        n261 = Add(x=w481, y=w476) -> (x+y=w480:dbl)
        n262 = Index Array(array=w474, index (col)=w480) -> (element=→"Feature extraction scan":dbl[])  [unwired: 1 in]
        n263 = call <vilib>:"3D Surface.vi"("z matrix"=w474, "3D graph"="3D Surface") -> ()  [unwired: 8 in, 2 out]
        n264 = local read "Completed"() -> (w482:bool)
        n265 = local read "Exit"() -> (w485:bool)
        n266 = Compound Arithmetic op=OR(w482, w485) -> (w484:bool)
        n267 = Wait Until Next ms Multiple(millisecond multiple=u32 100 ("ms 배수")) -> ()  [unwired: 1 out]
      }
      n268 = Release Queue(queue=w427) -> ()  [unwired: 2 in, 3 out]
      n269 = while {
        stop <- w459 stop-if-true
        n270 = event shown="[0] \"Plot style\", \"ViewMode\": Value Change" {
          selector: _ -> [_ _ _]
          dyn-events: _ -> [_ _ _]
          timeout: _ -> [_ _ _]
          tunnel: [_ w463 _] -> w459
          event "Plot style", "ViewMode": Value Change {
            n271 = event-data() -> ()  [unwired: 1 in, 2 out]
            n272 = local read "3D Surface"() -> (w462:refnum<k7>)
            n273 = property class="CWGraph3D"(reference=w462, "ViewMode"="ViewMode") -> ()  [unwired: 1 in, 2 out]
            n274 = call <vilib>:"Basic Properties.vi"("3D graph"=w462, "plot style"="Plot style") -> ()  [unwired: 12 in, 2 out]
          }
          event "Exit": Value Change {
            n275 = event-data() -> ()  [unwired: 1 in, 1 out]
            n276 = local read "Exit"() -> (w463:bool)
          }
          event "Max", "Min", "ColorMapAutoScale": Value Change {
            n277 = event-data() -> ()  [unwired: 1 in, 5 out]
            n278 = local read "3D Surface"() -> (w464:refnum<k7>)
            n279 = call "Surface_ColorScale.vi"("ColorMapAutoScale"="ColorMapAutoScale", "Min"="Min", "Max"="Max", "3D Surface_"=w464) -> ("Min 2"=w468:dbl, "Max 2"=w467:dbl)  [unwired: 1 in, 2 out]
            n280 = local write "Max"(w467) -> ()
            n281 = local write "Min"(w468) -> ()
          }
        }
      }
      n282 = TDMS Close(8:w435, 11:w436) -> (0:w433:errorcluster)  [unwired: 1 out]
      n283 = call <vilib>:"Simple Error Handler.vi"("error in (no error)"=w433) -> ()  [unwired: 2 in, 7 out]
      n284 = Release Queue(queue=w431) -> ()  [unwired: 2 in, 3 out]
      n285 = while {
        tunnel: w426 -> [w472]
        stop <- w471 stop-if-true
        n286 = call "CSV Save.vi"("Array"=w472, "Save Button"="Save Scan mode") -> ()  [unwired: 9 in, 1 out]
        n287 = Wait Until Next ms Multiple(millisecond multiple=u32 100 ("ms 배수")) -> ()  [unwired: 1 out]
        n288 = local read "Exit"() -> (w471:bool)
      }
    }
    frame "Lift-Off" {
      n289 = while {
        shift-right: [w711] -> _
        shift-left: "2D Array In" -> [w712]
        stop <- w716 stop-if-true
        n290 = call "CSV Open.vi"("2D Array In"=w712, "Open"="Open") -> ("2D Array Out"=w711:dbl[][])  [unwired: 9 in]
        n291 = Delete From Array(array=w711, index (col)=0 ("disabled index (col)")) -> (array with subset deleted=w713:dbl[][])  [unwired: 2 in, 1 out]
        n292 = Subtract(x=w713, y=w711) -> (x-y=w709:dbl[][])
        n293 = Transpose 2D Array(2D array=w709) -> (transposed array=w706:dbl[][])
        n294 = call "Filter_Lowpass - 2D.vi"("Filter"="Filter lf", "Input 2D"=w706, "low cutoff freq: fl"="Low cutoff freq: fl") -> ("Output"=w708:dbl[][])  [unwired: 6 in]
        n295 = Transpose 2D Array(2D array=w708) -> (transposed array=w705:dbl[][])
        n296 = Select(t=w705, s="View Mode", f=w711) -> (s? t:f=→"Hall sensors signal lf":dbl[][])
        n297 = local read "Exit"() -> (w716:bool)
      }
    }
    frame "                    Test mode                   " {
      n298 = call "tcp_init.vi"("port"=u16 8089) -> ("error out"=w717:errorcluster, "output cluster"=w718:T9)  [unwired: 9 in]
      n299 = while {
        tunnel: w733 -> [w759]
        tunnel: w729 -> [w758]
        tunnel: [w776] -> w731
        tunnel: [w777] -> w732
        shift-right: [w772] -> _
        shift-left: w730 -> [w773]
        tunnel: w730 -> [w771]
        shift-right: [w769] -> _
        shift-left: _ -> [w768]
        tunnel: w728 -> [w767]
        shift-right: [w766] -> _
        shift-left: _ -> [w765]
        shift-right: [w763] -> _
        shift-left: 1 ("Average") -> [w762]
        tunnel: w726 -> [w755]
        tunnel: w725 -> [w754]
        tunnel: w724 -> [w753]
        tunnel: w723 -> [w749]
        shift-right: [w744] -> _
        shift-left: dbl[][] [] -> [w745]
        shift-right: [w739] -> _
        shift-left: dbl[] [] -> [w738]
        shift-right: [w736] -> _
        shift-left: w717 -> [w734]
        shift-right: [w737] -> w719
        shift-left: w718 -> [w735]
        stop <- w778 stop-if-true
        n300 = First Call?() -> (First Call?: T/F=w760:bool)
        n301 = case shown="True" w760 {
          tunnel: w759 -> [w779 w784]
          tunnel: w758 -> [w780 w783]
          tunnel: [w779 w782] -> w757
          tunnel: [w780 w781] -> w756
          frame False {
          }
          frame True {
            n302 = call <vilib>:"DAQmx Start Task.vi"("task/channels in"=w784, "error in"=w783) -> ("task out"=w782:refnum<k21>, "error out"=w781:errorcluster)  [unwired: 12 in]
          }
        }
        n303 = local read "Pulser Cycles"() -> (w761:i32)
        n304 = call-poly <vilib>:"DAQmx Read.vi"("task/channels in"=w757, "number of samples per channel"=w749, "error in"=w756) -> ("task out"=w777:refnum<k21>, "data"=w748:waveform(dbl)[], "error out"=w776:errorcluster)  [unwired: 10 in]
        n305 = Quotient & Remainder(x=w762, y=w761) -> (x-y*floor(x/y)=w774:i32)  [unwired: 1 out]
        n306 = Equal To 0?(x=w774) -> (x = 0?=w752:bool)
        n307 = Index Array(array=w748, index #1=0 ("index (row)"), index #2=1 ("index")) -> (element #1=w750:waveform(dbl), element #2=w746:waveform(dbl))
        n308 = Unbundle By Name(w750) -> ("Y"=w740:dbl[])
        n309 = Add Array Elements(numeric array=w740) -> (sum=w742:dbl)
        n310 = Array Size(array=w740) -> (size(s)=w741:i32)
        n311 = Divide(x=w742, y=w741) -> (x/y=w743:dbl)
        n312 = Subtract(x=w740, y=w743) -> ()  [unwired: 1 out]
        n313 = Add(x=w740, y=w773) -> (x+y=w770:dbl[])
        n314 = case shown="False" w752 {
          tunnel: w761 -> [_ w835]
          tunnel: w750 -> [_ w831]
          tunnel: w770 -> [w793 w840]
          tunnel: [w793 w839] -> w772
          tunnel: w771 -> [_ w839]
          tunnel: [w792 w813] -> w769
          tunnel: w768 -> [w792 w838]
          tunnel: w767 -> [_ w826]
          tunnel: [w791 w836] -> w766
          tunnel: w765 -> [w791 w837]
          tunnel: [w789 1 ("Average")] -> w763
          tunnel: w762 -> [w790 _]
          tunnel: w755 -> [_ w827]
          tunnel: w754 -> [_ w829]
          tunnel: w753 -> [_ w828]
          tunnel: w746 -> [_ _]
          tunnel: [w788 w820] -> w744
          tunnel: w745 -> [w788 w819]
          tunnel: [w787 w805] -> w739
          tunnel: w738 -> [w787 w804]
          tunnel: w735 -> [w786 w797]
          tunnel: w734 -> [w785 w796]
          tunnel: [w786 w795] -> w737
          tunnel: [w785 w794] -> w736
          frame False {
            n315 = Increment(x=w790) -> (x+1=w789:i32)
          }
          frame True {
            n316 = Divide(x=w840, y=w835) -> (x/y=w803:dbl[])
            n317 = call "PECT_Feature extraction.vi"("Length T/2"=w826, "Offset"="Offset", "Length"=w827, "Start 2"=w828, "Start 1"=w829, "Pulse signal in"=w803) -> ()  [unwired: 5 in, 1 out]
            n318 = case shown="True" "Backdata" {
              tunnel: w803 -> [w848 w851]
              tunnel: [w848 w849] -> w805
              tunnel: w804 -> [_ w849]
              tunnel: [w848 w850] -> w800
              frame False {
              }
              frame True {
                n319 = Subtract(x=w851, y=w849) -> (x-y=w850:dbl[])
              }
            }
            n320 = call "Filter_Lowpass.vi"("Filter"="Filter 2", "Pulse signal in"=w800, "low cutoff freq: fl"="low cutoff freq: fl 2") -> ("Signal out"=w798:dbl[])  [unwired: 6 in]
            n321 = case shown="True" TRUE {
              tunnel: w798 -> [_ w843]
              tunnel: w797 -> [w842 w847]
              tunnel: w796 -> [w841 w846]
              tunnel: [w842 w845] -> w795
              tunnel: [w841 w844] -> w794
              frame False {
              }
              frame True {
                n322 = call "tcp_senddata.vi"("error In"=w846, "array"=w843, "Data In"=w847) -> ("Error Out"=w844:errorcluster, "Data Out"=w845:T9)  [unwired: 6 in, 1 out]
              }
            }
            n323 = Bundle By Name(cluster=w831, "Y"=w798) -> (w812:waveform(dbl))
            n324 = call-poly <vilib>:"FFT Power Spectrum and PSD.vi"("time signal"=w812) -> ("Power Spectrum / PSD"=w811:cluster{"f0":dbl, "df":dbl, "magnitude":dbl[]})  [unwired: 7 in, 3 out]
            n325 = case shown="True" "2 Plots" {
              tunnel: [w859 w865] -> w807
              tunnel: w838 -> [_ w864]
              tunnel: [w856 w864] -> w813
              tunnel: w812 -> [w856 w860]
              tunnel: w811 -> [w857 w862]
              tunnel: [w858 w863] -> w832
              tunnel: w837 -> [_ w861]
              tunnel: [w857 w861] -> w836
              frame False {
                n326 = Build Array(w857, w857) -> (w858:cluster{"f0":dbl, "df":dbl, "magnitude":dbl[]}[])
                n327 = Build Array(w856, w856) -> (w859:waveform(dbl)[])
              }
              frame True {
                n328 = Build Array(w861, w862) -> (w863:cluster{"f0":dbl, "df":dbl, "magnitude":dbl[]}[])
                n329 = Build Array(w864, w860) -> (w865:waveform(dbl)[])
              }
            }
            "Power spectral density" <- w832
            "Hall sensors signal" <- w807
            n330 = case shown="True" "Add LF" {
              tunnel: w798 -> [_ w855]
              tunnel: [w852 w853] -> w820
              tunnel: w819 -> [w852 w854]
              frame False {
              }
              frame True {
                n331 = Build Array (concatenate)(w854, w855) -> (w853:dbl[][])
              }
            }
            n332 = call "CSV Save.vi"("Array"=w820, "Save Button"="Save LF") -> ()  [unwired: 9 in, 1 out]
            n333 = Subtract(x="End idx", y="Start idx") -> (x-y=w814:i32)
            n334 = Array Subset(array=w798, index="Start idx", length=w814) -> (w809:dbl[])
            n335 = Square(x=w809) -> (x^2=w808:dbl[])
            n336 = Delete From Array(array=w820, index (col)=0 ("disabled index (col)")) -> (array with subset deleted=w821:dbl[][])  [unwired: 2 in, 1 out]
            n337 = Array Size(array=w809) -> (size(s)=w817:i32)
            n338 = Add Array Elements(numeric array=w808) -> (sum=w818:dbl)
            n339 = Divide(x=w818, y=w817) -> (x/y=→"Feature Extraction":dbl)
            n340 = Subtract(x=w821, y=w820) -> (x-y=→"dy":dbl[][])
          }
        }
        n341 = local read "Exit"() -> (w764:bool)
        n342 = Unbundle By Name(w776) -> ("status"=w775:bool)
        n343 = Or(x=w775, y=w764) -> (x .or. y?=w778:bool)
      }
      n344 = call "tcp_stop.vi"("Data"=w719) -> ()  [unwired: 11 in]
    }
  }
  n345 = VISA Close(VISA resource name=w41, error in (no error)=w40) -> (error out=w38:errorcluster)
  n346 = VISA Close(VISA resource name=w42, error in (no error)=w43) -> (error out=w39:errorcluster)
  n347 = call <vilib>:"Simple Error Handler.vi"("error in (no error)"=w38) -> ()  [unwired: 4 in, 5 out]
  n348 = call <vilib>:"Simple Error Handler.vi"("error in (no error)"=w39) -> ()  [unwired: 4 in, 5 out]
  n349 = while {
    shift-right: [w886] -> _
    shift-left: T1."No Scan" -> [w891]
    shift-right: [w882] -> _
    shift-left: 0.0 ("Current  Position (mm)") -> [w890]
    shift-right: [w883] -> _
    shift-left: 0.0 ("Current  Position (mm)") -> [w889]
    shift-right: [w881] -> _
    shift-left: 0.0 ("Current  Position (mm)") -> [w888]
    shift-right: [w880] -> _
    shift-left: 0.0 ("Current  Position (mm)") -> [w887]
    tunnel: w28 -> [w885]
    tunnel: w27 -> [w872]
    tunnel: w30 -> [w884]
    tunnel: w29 -> [w871]
    tunnel: [w879] -> _
    tunnel: [w877] -> w36
    tunnel: [w878] -> _
    tunnel: [w876] -> w37
    shift-right: [w869] -> _
    shift-left: 0.0 ("Current  Position (mm)") -> [w868]
    stop <- w873 stop-if-true
    n350 = case shown="\"Wait X\"" w891 {
      selector: w891 -> [w910 _ _ _ _]
      tunnel: w890 -> [w903 w970 w992 w1056 w1096]
      tunnel: w889 -> [w904 w969 w998 w1055 w1095]
      tunnel: w888 -> [_ w968 w1015 w1036 w1079]
      tunnel: w887 -> [_ w967 w1016 w1054 w1077]
      tunnel: [w909 T1."Wait X" w994 w1047 w1081] -> w886
      tunnel: w885 -> [w908 w962 w1011 w1045 w1090]
      tunnel: w872 -> [w907 w963 w1012 w1046 w1091]
      tunnel: w884 -> [w906 w964 w1004 w1041 w1093]
      tunnel: w871 -> [w905 w965 w1005 w1042 w1092]
      tunnel: [w896 w969 w998 w1055 w1095] -> w883
      tunnel: [w895 w970 w995 w1056 w1096] -> w882
      tunnel: [w898 w968 w1015 w1036 w1094] -> w881
      tunnel: [w897 w967 w1016 w1054 w1077] -> w880
      tunnel: [w902 w956 w1009 w1044 w1088] -> w879
      tunnel: [w901 w955 w1007 w1043 w1086] -> w877
      tunnel: [w900 w954 w1013 w1039 w1084] -> w878
      tunnel: [w899 w953 w1014 w1040 w1082] -> w876
      tunnel: w872 -> [_ _ _ _ _]
      tunnel: [w894 w952 w985 w1034 w1073] -> w869
      tunnel: w868 -> [w893 w952 w991 w1034 w1073]
      frame "No Scan", Default {
        n351 = local read "Scan"() -> (w892:bool)
        n352 = case shown="True" w892 {
          tunnel: w910 -> [w918 _]
          tunnel: [w918 w929] -> w909
          tunnel: w908 -> [w915 w927]
          tunnel: w907 -> [w916 w926]
          tunnel: w906 -> [w913 w925]
          tunnel: w905 -> [w914 w924]
          tunnel: w904 -> [w912 _]
          tunnel: w903 -> [w917 _]
          tunnel: [w917 w923] -> w895
          tunnel: [w916 w933] -> w902
          tunnel: [w915 w932] -> w901
          tunnel: [w914 w931] -> w900
          tunnel: [w913 w930] -> w899
          tunnel: [w912 w928] -> w898
          tunnel: [w911 w923] -> w894
          tunnel: w893 -> [w911 _]
          frame False {
          }
          frame True {
            n353 = flat-sequence {
              tunnel: w924 -> [w934]
              tunnel: w925 -> [w935]
              tunnel: w926 -> [w936]
              tunnel: w927 -> [w937]
              tunnel: [w937] -> w922
              tunnel: [w936] -> w921
              tunnel: [w935] -> w920
              tunnel: [w934] -> w919
              tunnel: [w951] -> w933
              tunnel: [w950] -> w932
              tunnel: [w949] -> w931
              tunnel: [w948] -> w930
              tunnel: [T1."Move X"] -> w929
              tunnel: [w946] -> w928
              tunnel: [w939] -> w923
              tunnel: w922 -> [w945]
              tunnel: w921 -> [w944]
              tunnel: w920 -> [w943]
              tunnel: w919 -> [w942]
              frame #0 {
              }
              frame #1 {
                n354 = local write "Direction (+)"("+" ("Direction (+)")) -> ()
                n355 = local write "Numeric"(0.0 ("Numeric")) -> ()
                n356 = local read "Travel per Pulse (mm)"() -> (w941:dbl)
                n357 = call "Autonics_GetPos.vi"("error in (no error)"=w945, "Travel per Pulse (mm)"=w941, "VISA resource name"=w944) -> ("error out"=w950:errorcluster, "Current  Position (mm)"=w939:dbl, "VISA resource name out"=w951:refnum<visa-resource-name>)  [unwired: 6 in]
                "Start Pos Y" <- w939
                n358 = call "Autonics_GetPos.vi"("error in (no error)"=w943, "Travel per Pulse (mm)"=w941, "VISA resource name"=w942) -> ("error out"=w948:errorcluster, "Current  Position (mm)"=w946:dbl, "VISA resource name out"=w949:refnum<visa-resource-name>)  [unwired: 6 in]
                "Start Pos X" <- w946
                n359 = local write "Cur. Pos X"(w939) -> ()
                n360 = local write "Cur. Pos Y"(w946) -> ()
              }
            }
          }
        }
        n361 = local read "X - length"() -> (w896:dbl)
        n362 = local read "Step Y"() -> (w897:dbl)
      }
      frame "Move X" {
        n363 = local read "Travel per Pulse (mm)"() -> (w957:dbl)
        n364 = local read "X - length"() -> (w958:dbl)
        n365 = call "Autonics_Move.vi"("Direction (+)"="Direction (+)", "error in (no error)"=w962, "Travel per Pulse (mm)"=w957, "Move Distance (mm)"=w958, "VISA resource name"=w963) -> ("error out"=w960:errorcluster, "VISA resource name out"=w961:refnum<visa-resource-name>)  [unwired: 5 in]
        n366 = flat-sequence {
          tunnel: [w975] -> w956
          tunnel: w961 -> [w975]
          tunnel: [w974] -> w955
          tunnel: w960 -> [w974]
          tunnel: [w972] -> w954
          tunnel: w965 -> [w972]
          tunnel: [w971] -> w953
          tunnel: w964 -> [w971]
          frame #0 {
            n367 = Wait (ms)(milliseconds to wait=u32 100) -> ()  [unwired: 1 out]
          }
        }
      }
      frame "Wait X" {
        n368 = local read "Travel per Pulse (mm)"() -> (w1002:dbl)
        n369 = call "Autonics_GetPos.vi"("error in (no error)"=w1004, "Travel per Pulse (mm)"=w1002, "VISA resource name"=w1005) -> ("error out"=w1003:errorcluster, "Current  Position (mm)"=w1001:dbl, "VISA resource name out"=w1006:refnum<visa-resource-name>)  [unwired: 6 in]
        n370 = call "Autonics_GetPos.vi"("error in (no error)"=w1011, "Travel per Pulse (mm)"=w1002, "VISA resource name"=w1012) -> ("error out"=w1008:errorcluster, "Current  Position (mm)"=w983:dbl, "VISA resource name out"=w1010:refnum<visa-resource-name>)  [unwired: 6 in]
        n371 = local read "Direction (+)"() -> (w978:string)
        n372 = local write "Cur. Pos Y"(w1001) -> ()
        n373 = Equal?(x=w978, y="-") -> (x = y?=w976:bool)
        n374 = local read "Step X"() -> (w988:dbl)
        n375 = local write "Cur. Pos X"(w983) -> ()
        n376 = Subtract(x=w983, y=w991) -> (x-y=w990:dbl)
        n377 = Absolute Value(x=w998) -> (abs(x)=w1000:dbl)
        n378 = Absolute Value(x=w990) -> (abs(x)=w989:dbl)
        n379 = Subtract(x=w983, y=w992) -> (x-y=w999:dbl)
        n380 = Greater Or Equal?(x=w989, y=w988) -> (x >= y?=w984:bool)
        n381 = Quotient & Remainder(x=w983, y=w988) -> (floor(x/y)=w980:dbl)  [unwired: 1 out]
        n382 = Absolute Value(x=w999) -> (abs(x)=w993:dbl)
        n383 = Subtract(x=w993, y=w1000) -> (x-y=w996:dbl)
        n384 = case shown="True" w984 {
          selector: w984 -> [_ w1017]
          frame False {
          }
          frame True {
            n385 = local read "Numeric"() -> (w1019:dbl)
            n386 = Increment(x=w1019) -> (x+1=→"Numeric":dbl)
            "Acquire" <- w1017
          }
        }
        n387 = Increment(x=w980) -> (x+1=w981:dbl)
        n388 = call "Convert Double Precision.vi"("Input"=w996) -> ("Output"=w997:dbl)  [unwired: 10 in]
        n389 = Select(t=w981, s=w976, f=w980) -> (s? t:f=w979:dbl)
        n390 = Multiply(x=w979, y=w988) -> (x*y=w987:dbl)
        n391 = Select(t=w987, s=w984, f=w991) -> (s? t:f=w986:dbl)
        n392 = Greater Or Equal To 0?(x=w997) -> (x >= 0?=w982:bool)
        n393 = Select(t=w983, s=w982, f=w986) -> (s? t:f=w985:dbl)
        n394 = case shown="True" w982 {
          tunnel: [w1022 w1033] -> w1014
          tunnel: w1003 -> [w1022 w1033]
          tunnel: [w1023 w1032] -> w1013
          tunnel: w1006 -> [w1023 w1032]
          tunnel: [w1025 w1031] -> w1009
          tunnel: w1010 -> [w1025 w1031]
          tunnel: [w1024 w1030] -> w1007
          tunnel: w1008 -> [w1024 w1030]
          tunnel: [w1021 w1029] -> w995
          tunnel: w992 -> [w1021 _]
          tunnel: [T1."Wait X" T1."Move Y"] -> w994
          frame False {
          }
          frame True {
            n395 = local read "Cur. Pos X"() -> (w1029:dbl)
            n396 = local write "Numeric"(0.0 ("Numeric")) -> ()
            n397 = Wait (ms)(milliseconds to wait=u32 1000) -> ()  [unwired: 1 out]
          }
        }
        "Current  Position (mm)" <- w991
      }
      frame "Move Y" {
        n398 = local read "Step Y"() -> (w1050:dbl)
        n399 = local read "Y - length"() -> (w1035:dbl)
        n400 = local read "Start Pos Y"() -> (w1037:dbl)
        n401 = Subtract(x=w1035, y=w1050) -> ()  [unwired: 1 out]
        n402 = Subtract(x=w1037, y=w1036) -> (x-y=w1053:dbl)
        n403 = Absolute Value(x=w1035) -> (abs(x)=w1051:dbl)
        n404 = Absolute Value(x=w1053) -> (abs(x)=w1052:dbl)
        n405 = Subtract(x=w1052, y=w1051) -> (x-y=w1049:dbl)
        n406 = call "Convert Double Precision.vi"("Input"=w1049) -> ("Output"=w1048:dbl)  [unwired: 10 in]
        n407 = Greater Or Equal To 0?(x=w1048) -> (x >= 0?=w1038:bool)
        n408 = case shown="True" w1038 {
          tunnel: [T1."Wait Y" T1."No Scan"] -> w1047
          tunnel: w1046 -> [w1064 w1070]
          tunnel: [w1065 w1069] -> w1043
          tunnel: w1045 -> [w1065 w1069]
          tunnel: [w1064 w1070] -> w1044
          tunnel: w1042 -> [w1058 w1068]
          tunnel: w1041 -> [w1062 w1067]
          tunnel: [w1063 w1067] -> w1040
          tunnel: [w1057 w1068] -> w1039
          frame False {
            n409 = local read "Step Y"() -> (w1061:dbl)
            n410 = local read "Travel per Pulse (mm)"() -> (w1059:dbl)
            n411 = call "Autonics_Move.vi"("Direction (+)"="+" ("Direction (+) 2"), "error in (no error)"=w1062, "Travel per Pulse (mm)"=w1059, "Move Distance (mm)"=w1061, "VISA resource name"=w1058) -> ("error out"=w1063:errorcluster, "VISA resource name out"=w1057:refnum<visa-resource-name>)  [unwired: 5 in]
          }
          frame True {
            n412 = local write "Scan"(FALSE) -> ()
          }
        }
      }
      frame "Wait Y" {
        n413 = local read "Travel per Pulse (mm)"() -> (w1074:dbl)
        n414 = call "Autonics_GetPos.vi"("error in (no error)"=w1093, "Travel per Pulse (mm)"=w1074, "VISA resource name"=w1092) -> ("error out"=w1083:errorcluster, "Current  Position (mm)"=w1078:dbl, "VISA resource name out"=w1085:refnum<visa-resource-name>)  [unwired: 6 in]
        n415 = call "Autonics_GetPos.vi"("error in (no error)"=w1090, "Travel per Pulse (mm)"=w1074, "VISA resource name"=w1091) -> ("error out"=w1087:errorcluster, "Current  Position (mm)"=w1080:dbl, "VISA resource name out"=w1089:refnum<visa-resource-name>)  [unwired: 6 in]
        n416 = Subtract(x=w1078, y=w1079) -> (x-y=w1098:dbl)
        n417 = Absolute Value(x=w1077) -> (abs(x)=w1100:dbl)
        n418 = Absolute Value(x=w1098) -> (abs(x)=w1099:dbl)
        n419 = Subtract(x=w1099, y=w1100) -> (x-y=w1097:dbl)
        n420 = local write "Cur. Pos X"(w1080) -> ()
        n421 = local write "Cur. Pos Y"(w1078) -> ()
        n422 = call "Convert Double Precision.vi"("Input"=w1097) -> ("Output"=w1076:dbl)  [unwired: 10 in]
        n423 = Greater Or Equal To 0?(x=w1076) -> (x >= 0?=w1075:bool)
        n424 = case shown="True" w1075 {
          tunnel: w1079 -> [w1106 _]
          tunnel: [w1106 w1119] -> w1094
          tunnel: w1089 -> [w1105 w1117]
          tunnel: [w1105 w1117] -> w1088
          tunnel: [w1104 w1116] -> w1086
          tunnel: w1087 -> [w1104 w1116]
          tunnel: [w1103 w1115] -> w1084
          tunnel: w1085 -> [w1103 w1115]
          tunnel: [w1102 w1114] -> w1082
          tunnel: w1083 -> [w1102 w1114]
          tunnel: [T1."Wait Y" T1."Move X"] -> w1081
          frame False {
          }
          frame True {
            n425 = local read "Direction (+)"() -> (w1113:string)
            n426 = local read "Cur. Pos Y"() -> (w1119:dbl)
            n427 = Equal?(x=w1113, y="+") -> (x = y?=w1111:bool)
            n428 = Select(t="-", s=w1111, f="+") -> (s? t:f=w1110:string)
            n429 = local write "Direction (+)"(w1110) -> ()
            n430 = Wait (ms)(milliseconds to wait=u32 1000) -> ()  [unwired: 1 out]
          }
        }
      }
    }
    n431 = Wait Until Next ms Multiple(millisecond multiple=u32 100 ("milliseconds to wait")) -> ()  [unwired: 1 out]
    n432 = local read "Completed"() -> (w867:bool)
    n433 = local read "Exit"() -> (w866:bool)
    n434 = Unbundle By Name(w876) -> ("status"=w874:bool)
    n435 = Unbundle By Name(w877) -> ("status"=w875:bool)
    n436 = Compound Arithmetic op=OR(w867, w866, w875, w874) -> (w873:bool)
    "Enum" <- w891
  }
  n437 = call <vilib>:"DAQmx Clear Task.vi"("task in"=w91, "error in"=w90) -> ("error out"=w97:errorcluster)  [unwired: 13 in]
  n438 = call <vilib>:"Simple Error Handler.vi"("error in (no error)"=w97) -> ()  [unwired: 4 in, 5 out]
  n439 = call <vilib>:"Simple Error Handler.vi"("error in (no error)"=w36) -> ()  [unwired: 4 in, 5 out]
  n440 = call <vilib>:"Simple Error Handler.vi"("error in (no error)"=w37) -> ()  [unwired: 4 in, 5 out]
  n441 = call <vilib>:"Simple Error Handler.vi"() -> ()  [unwired: 5 in, 5 out]
